vi "Executor_v2.vi"() -> ()   [LabVIEW 2018]
uses:
  QBuilder Files/Actions_arr.ctl
  QBuilder Files/Action.ctl
  QBuilder Files/Parameters.ctl
  Executor Files/MacroInfo.ctl
  Executor Files/Calibrations.ctl
  Executor Files/VariableScan_Cluster.ctl
  Executor Files/RT Actions.ctl
  Executor Files/RT/ActionCluster.ctl
  Executor Files/RT/Instructions_RT.ctl
  Executor Files/RT/ParameterSubCluster.ctl
  Executor Files/State.ctl
  <vilib>/NI/AMC/Message Queue.ctl
  <vilib>/NI/AMC/Message.ctl
  <vilib>/NI/Tools/Keyed Array/KeyedArray.ctl
  Executor Files/RT/Target/Request.ctl
  <vilib>/NI/AMC/Create Single Message.vi
  <vilib>/NI/AMC/Update Message Routing Info.vi
  <vilib>/NI/AMC/Read Termination Message.vi
  <vilib>/NI/AMC/Send Message.vi
  <vilib>/NI/AMC/Globals.vi
  <vilib>/NI/AMC/AMC.lvlib
  <vilib>/NI/Tools/Keyed Array/Tools_KeyedArray.lvlib
panel:
  out "State":T1=enum."idle"
  out "Times (ms)":i64[](array[numeric])
  in  "System":u16(ring)=1 items=["Cusp", "Positron", "Musashi"]
  out "# always zero":i32
  out "error out":errorcluster
  in  "Macro Info 2D":T2(array[cluster])=[[{"Duration (s)"=0.1, "Instruction Description"="", "Input Bits"=[], "Output Bits"=[FALSE, FALSE, FALSE, FALSE, FALSE, FALSE, FALSE, FALSE, FALSE, FALSE, FALSE, FALSE, FALSE, FALSE, FALSE, FALSE, FALSE, FALSE, FALSE, FALSE, FALSE, FALSE, FALSE, FALSE, FALSE, FALSE, FALSE, FALSE, FALSE, FALSE, FALSE, FALSE, FALSE, FALSE, FALSE, FALSE, FALSE, FALSE], "Excitations"=[0.0, 0.0, 0.0, 0.0, 0.0, 0.0, 0.0, 0.0, 0.0, 0.0, 0.0, 0.0, 0.0, 0.0, 0.0, 0.0, 0.0, 0.0, 0.0, 0.0, 0.0, 0.0, 0.0, 0.0], "Steps"=1, "Changes"=[TRUE, TRUE]}, {"Duration (s)"=0.0, "Instruction Description"="", "Input Bits"=[], "Output Bits"=[], "Excitations"=[], "Steps"=0, "Changes"=[]}, {"Duration (s)"=0.0, "Instruction Description"="", "Input Bits"=[], "Output Bits"=[], "Excitations"=[], "Steps"=0, "Changes"=[]}, {"Duration (s)"=0.0, "Instruction Description"="", "Input Bits"=[], "Output Bits"=[], "Excitations"=[], "Steps"=0, "Changes"=[]}], [{"Duration (s)"=0.2, "Instruction Description"="", "Input Bits"=[], "Output Bits"=[FALSE, FALSE, FALSE, FALSE, FALSE, FALSE, FALSE, FALSE, FALSE, FALSE, FALSE, FALSE, FALSE, FALSE, FALSE, FALSE, FALSE, FALSE, FALSE, FALSE, FALSE, FALSE, FALSE, FALSE, FALSE, FALSE, FALSE, FALSE, FALSE, FALSE, FALSE, FALSE, FALSE, FALSE, FALSE, FALSE, FALSE, FALSE], "Excitations"=[0.0, 0.0, 0.0, 0.0, 0.0, 0.0, 0.0, 0.0, 0.0, 0.0, 0.0, 0.0, 0.0, 0.0, 0.0, 0.0, 0.0, 0.0, 0.0, 0.0, 0.0, 0.0, 0.0, 0.0], "Steps"=1, "Changes"=[TRUE, TRUE]}, {"Duration (s)"=0.0, "Instruction Description"="", "Input Bits"=[], "Output Bits"=[], "Excitations"=[], "Steps"=0, "Changes"=[]}, {"Duration (s)"=0.0, "Instruction Description"="", "Input Bits"=[], "Output Bits"=[], "Excitations"=[], "Steps"=0, "Changes"=[]}, {"Duration (s)"=0.0, "Instruction Description"="", "Input Bits"=[], "Output Bits"=[], "Excitations"=[], "Steps"=0, "Changes"=[]}], [{"Duration (s)"=0.3, "Instruction Description"="", "Input Bits"=[], "Output Bits"=[FALSE, FALSE, FALSE, FALSE, FALSE, FALSE, FALSE, FALSE, FALSE, FALSE, FALSE, FALSE, FALSE, FALSE, FALSE, FALSE, FALSE, FALSE, FALSE, FALSE, FALSE, FALSE, FALSE, FALSE, FALSE, FALSE, FALSE, FALSE, FALSE, FALSE, FALSE, FALSE, FALSE, FALSE, FALSE, FALSE, FALSE, FALSE], "Excitations"=[0.0, 0.0, 0.0, 0.0, 0.0, 0.0, 0.0, 0.0, 0.0, 0.0, 0.0, 0.0, 0.0, 0.0, 0.0, 0.0, 0.0, 0.0, 0.0, 0.0, 0.0, 0.0, 0.0, 0.0], "Steps"=1, "Changes"=[TRUE, TRUE]}, {"Duration (s)"=0.0, "Instruction Description"="", "Input Bits"=[], "Output Bits"=[], "Excitations"=[], "Steps"=0, "Changes"=[]}, {"Duration (s)"=0.0, "Instruction Description"="", "Input Bits"=[], "Output Bits"=[], "Excitations"=[], "Steps"=0, "Changes"=[]}, {"Duration (s)"=0.0, "Instruction Description"="", "Input Bits"=[], "Output Bits"=[], "Excitations"=[], "Steps"=0, "Changes"=[]}], [{"Duration (s)"=0.01, "Instruction Description"="", "Input Bits"=[], "Output Bits"=[FALSE, FALSE, FALSE, FALSE, FALSE, FALSE, FALSE, FALSE, FALSE, FALSE, FALSE, FALSE, FALSE, FALSE, FALSE, FALSE, FALSE, FALSE, FALSE, FALSE, FALSE, FALSE, FALSE, FALSE, FALSE, FALSE, FALSE, FALSE, FALSE, FALSE, FALSE, FALSE, FALSE, FALSE, FALSE, FALSE, FALSE, FALSE], "Excitations"=[-0.00023318098842089834, -0.00044019955713256676, -0.0004811194044810927, -0.0003270089360197006, -0.00037474988790963174, -0.00027444024231065297, 0.6717526466140145, -0.0003012834675718561, -0.0003574123346967952, -0.0002612820237967628, -0.00044389144836399103, -0.0003012330472735062, -0.00021413562815348174, -0.000348292029470864, -0.0006236629805725628, -0.0003687933751299158, -0.0009869232667160128, -0.00016073401868532967, -0.000402023518375825, -0.0002482954850485854, -0.0003689863609223317, -0.00026807315716459023, -8.725125004194771e-05, -0.00026778601219765283], "Steps"=1, "Changes"=[TRUE, FALSE]}, {"Duration (s)"=0.02, "Instruction Description"="", "Input Bits"=[], "Output Bits"=[FALSE, FALSE, FALSE, FALSE, FALSE, FALSE, FALSE, FALSE, FALSE, FALSE, FALSE, FALSE, FALSE, FALSE, FALSE, FALSE, FALSE, FALSE, FALSE, FALSE, FALSE, FALSE, FALSE, FALSE, FALSE, FALSE, FALSE, FALSE, FALSE, FALSE, FALSE, FALSE, FALSE, FALSE, FALSE, FALSE, FALSE, FALSE], "Excitations"=[-0.00023318098842089834, -0.00044019955713256676, -0.0004811194044810927, -0.0003270089360197006, -0.00037474988790963174, -0.00027444024231065297, 0.6717526466140145, -0.0003012834675718561, -0.0003574123346967952, -0.0002612820237967628, -0.00044389144836399103, -0.0003012330472735062, -0.00021413562815348174, -0.000348292029470864, -0.0006236629805725628, -0.0003687933751299158, -0.0009869232667160128, -0.00016073401868532967, -0.000402023518375825, -0.0002482954850485854, -0.0003689863609223317, -0.00026807315716459023, -8.725125004194771e-05, -0.00026778601219765283], "Steps"=100, "Changes"=[FALSE, TRUE]}, {"Duration (s)"=0.1, "Instruction Description"="wait", "Input Bits"=[], "Output Bits"=[FALSE, FALSE, FALSE, FALSE, FALSE, FALSE, FALSE, FALSE, FALSE, FALSE, FALSE, FALSE, FALSE, FALSE, FALSE, FALSE, FALSE, FALSE, FALSE, FALSE, FALSE, FALSE, FALSE, FALSE, FALSE, FALSE, FALSE, FALSE, FALSE, FALSE, FALSE, FALSE, FALSE, FALSE, FALSE, FALSE, FALSE, FALSE], "Excitations"=[-0.00023318098842089834, -0.00044019955713256676, -0.0004811194044810927, -0.0003270089360197006, -0.00037474988790963174, -0.00027444024231065297, 0.6717526466140145, -0.0003012834675718561, -0.0003574123346967952, -0.0002612820237967628, -0.00044389144836399103, -0.0003012330472735062, -0.00021413562815348174, -0.000348292029470864, -0.0006236629805725628, -0.0003687933751299158, -0.0009869232667160128, -0.00016073401868532967, -0.000402023518375825, -0.0002482954850485854, -0.0003689863609223317, -0.00026807315716459023, -8.725125004194771e-05, -0.00026778601219765283], "Steps"=1, "Changes"=[FALSE, FALSE]}, {"Duration (s)"=0.01, "Instruction Description"="wait", "Input Bits"=[], "Output Bits"=[FALSE, FALSE, FALSE, FALSE, FALSE, FALSE, FALSE, FALSE, FALSE, FALSE, FALSE, FALSE, FALSE, FALSE, FALSE, FALSE, FALSE, FALSE, FALSE, FALSE, FALSE, FALSE, FALSE, FALSE, FALSE, FALSE, FALSE, FALSE, FALSE, FALSE, FALSE, FALSE, FALSE, FALSE, FALSE, FALSE, FALSE, FALSE], "Excitations"=[-0.00023318098842089834, -0.00044019955713256676, -0.0004811194044810927, -0.0003270089360197006, -0.00037474988790963174, -0.00027444024231065297, -0.0004032935641068728, -0.0003012834675718561, -0.0003574123346967952, -0.0002612820237967628, -0.00044389144836399103, -0.0003012330472735062, -0.00021413562815348174, -0.000348292029470864, -0.0006236629805725628, -0.0003687933751299158, -0.0009869232667160128, -0.00016073401868532967, -0.000402023518375825, -0.0002482954850485854, -0.0003689863609223317, -0.00026807315716459023, -8.725125004194771e-05, -0.00026778601219765283], "Steps"=100, "Changes"=[FALSE, TRUE]}], [{"Duration (s)"=0.1, "Instruction Description"="", "Input Bits"=[], "Output Bits"=[FALSE, FALSE, FALSE, FALSE, FALSE, FALSE, FALSE, FALSE, FALSE, FALSE, FALSE, FALSE, FALSE, FALSE, FALSE, FALSE, FALSE, FALSE, FALSE, FALSE, FALSE, FALSE, FALSE, FALSE, FALSE, FALSE, FALSE, FALSE, FALSE, FALSE, FALSE, FALSE, FALSE, FALSE, FALSE, FALSE, FALSE, FALSE], "Excitations"=[-0.00023318098842089834, -0.00044019955713256676, -0.0004811194044810927, -0.0003270089360197006, -0.00037474988790963174, -0.00027444024231065297, -0.0004032935641068728, -0.0003012834675718561, -0.0003574123346967952, -0.0002612820237967628, -0.00044389144836399103, -0.0003012330472735062, -0.00021413562815348174, -0.000348292029470864, -0.0006236629805725628, -0.0003687933751299158, -0.0009869232667160128, -0.00016073401868532967, -0.000402023518375825, -0.0002482954850485854, -0.0003689863609223317, -0.00026807315716459023, -8.725125004194771e-05, -0.00026778601219765283], "Steps"=1, "Changes"=[TRUE, TRUE]}, {"Duration (s)"=0.0, "Instruction Description"="", "Input Bits"=[], "Output Bits"=[], "Excitations"=[], "Steps"=0, "Changes"=[]}, {"Duration (s)"=0.0, "Instruction Description"="", "Input Bits"=[], "Output Bits"=[], "Excitations"=[], "Steps"=0, "Changes"=[]}, {"Duration (s)"=0.0, "Instruction Description"="", "Input Bits"=[], "Output Bits"=[], "Excitations"=[], "Steps"=0, "Changes"=[]}]] {"Duration (s)" format="%_6p"; "Excitations" format="%_3f"}
  in  "stop":bool
  in  "Tab Control":T3(tab)
  in  "List Cycles":u32
  in  "Cycles":u32
  out "Ping":bool
  out "Sending":bool
  in  "Target stale":bool
  in  "Slave?":bool
  in  "Variable Scan":bool
  in  "Zero All":bool
  out "Time (s)":dbl=0.866 format="%.3f"
  out "% completed":dbl(slide)=1.0 scale=0.0..1.0
  out "Duration (s)":dbl=0.8660000000000001 format="%.3f"
  in  "Stale":bool
  in  "Run":bool
  out "Cue Description":string="a few lines of nothing"
  in  "Cue Path":path=path "C:/CuspControl/Positron/1_Cues/Test/2026-04-21/simple3.q"
  out "Cue Info":T4(array[cluster])=[{"Duration (s)"=0.1, "Action Description"=""}, {"Duration (s)"=0.2, "Action Description"=""}, {"Duration (s)"=0.3, "Action Description"=""}, {"Duration (s)"=0.144, "Action Description"="10 V, 0 V"}, {"Duration (s)"=0.1, "Action Description"=""}] {"Duration (s)" format="%_6p"}
  out "Current\nAction":i32
  in  "ABORT":bool
  in  "Favorites":T5(array[cluster])=[{"Cue Path"=path "C:/CuspControl/Positron/1_Cues/RealBaseline/FPS_1s.q", "Slave"=FALSE, "Cycle"=1, "Completed"=0}, {"Cue Path"=path "C:/CuspControl/Positron/1_Cues/RealBaseline/Stack_v23_mcp_1.q", "Slave"=FALSE, "Cycle"=1, "Completed"=0}, {"Cue Path"=path "C:/CuspControl/Positron/1_Cues/Baseline/Stack_v23_s_100.q", "Slave"=FALSE, "Cycle"=1, "Completed"=0}, {"Cue Path"=path "C:/CuspControl/Positron/1_Cues/Util/BiasModerator.q", "Slave"=FALSE, "Cycle"=1, "Completed"=0}]
  out "Timing":i64[](graph)=[104, 204, 304, 150, 104]
  in  "Skip wait":bool
  in  "Params deadtime (s)":dbl=0.004
  in  "Macro deadtime (s)":dbl=0.006
  out "RepAct#list":i32[](array[numeric])=[0, 1, 2, 3, 4]
  in  "# AO cards":u8=3
  out "# trodes\nin calibr":u8=24
  in  "Save Calibration":bool
  in  "Open Calibration":bool
  in  "Calibrations":T6=[{"Gain"=15.0098, "Offset (V)"=0.0035, "Name"="Vm"}, {"Gain"=14.9932, "Offset (V)"=0.0066, "Name"="in"}, {"Gain"=14.9651, "Offset (V)"=0.0072, "Name"="s1"}, {"Gain"=14.9843, "Offset (V)"=0.0049, "Name"="s2"}, {"Gain"=14.9433, "Offset (V)"=0.0056, "Name"="s3r"}, {"Gain"=14.9395, "Offset (V)"=0.0041, "Name"="s3s"}, {"Gain"=14.8775, "Offset (V)"=0.006, "Name"="s4"}, {"Gain"=14.9361, "Offset (V)"=0.0045, "Name"="g8"}, {"Gain"=15.1086, "Offset (V)"=0.0054, "Name"="e1"}, {"Gain"=14.9264, "Offset (V)"=0.0039, "Name"="c1"}, {"Gain"=14.8685, "Offset (V)"=0.0066, "Name"="c2"}, {"Gain"=14.9386, "Offset (V)"=0.0045, "Name"="c3"}, {"Gain"=14.9438, "Offset (V)"=0.0032, "Name"="c4"}, {"Gain"=14.93, "Offset (V)"=0.0052, "Name"="c5"}, {"Gain"=14.9119, "Offset (V)"=0.0093, "Name"="c6"}, {"Gain"=14.9135, "Offset (V)"=0.0055, "Name"="c7"}, {"Gain"=14.9961, "Offset (V)"=0.0148, "Name"="c8"}, {"Gain"=14.9315, "Offset (V)"=0.0024, "Name"="c9"}, {"Gain"=14.9245, "Offset (V)"=0.006, "Name"="e2"}, {"Gain"=14.9016, "Offset (V)"=0.0037, "Name"="--"}, {"Gain"=14.9057, "Offset (V)"=0.0055, "Name"="--"}, {"Gain"=14.9213, "Offset (V)"=0.004, "Name"="--"}, {"Gain"=14.8995, "Offset (V)"=0.0013, "Name"="--"}, {"Gain"=14.9373, "Offset (V)"=0.004, "Name"="--"}] {"Offset (V)" format="%_6p"; "Gain" format="%_6p"}
  in  "Calibration path":path=path "C:/CuspControl/Positron/Configuration/Calibration/Zz_Gal_to_Area.cal"
  out "# electrodes error":bool=TRUE
  in  "outbits (38)":i32=38
  in  "iswap1_1":i32
  in  "iswap1_2":i32
  in  "iswap2_1":i32
  in  "iswap2_2":i32
  in  "Tab Control 2":T7(tab)=enum."VI Server"
  out "Actions":T8=[{"Toggle"=TRUE, "Open parameter editor"=FALSE, "Open MacroEditor"=FALSE, "Macro path"=path "", "Duration (s)"=0.1, "Parameters"=[{"Status"="Camera", "Name"="state (0,1)", "Value"=0.0, "Changed"=FALSE}, {"Status"="Slave", "Name"="state (0,1)", "Value"=0.0, "Changed"=FALSE}, {"Status"="Wait", "Name"="inbit (0...7)", "Value"=0.0, "Changed"=FALSE}, {"Status"="Coils", "Name"="buncher (A)", "Value"=0.0, "Changed"=FALSE}, {"Status"="Coils", "Name"="michishio (A)", "Value"=0.0, "Changed"=FALSE}, {"Status"="Coils", "Name"="acorn (A)", "Value"=0.0, "Changed"=FALSE}, {"Status"="Coils", "Name"="stacker (A)", "Value"=0.0, "Changed"=FALSE}, {"Status"="Coils", "Name"="T2 + T3 (A)", "Value"=0.0, "Changed"=FALSE}, {"Status"="Coils", "Name"="T4 (A)  ", "Value"=0.0, "Changed"=FALSE}, {"Status"="Coils", "Name"="-------- (A)", "Value"=0.0, "Changed"=FALSE}, {"Status"="RW", "Name"="mode (0-9)", "Value"=0.0, "Changed"=FALSE}, {"Status"="RW", "Name"="f_start (Hz)", "Value"=0.0, "Changed"=FALSE}, {"Status"="RW", "Name"="f_stop (Hz)", "Value"=0.0, "Changed"=FALSE}, {"Status"="RW", "Name"="amplitude (V)", "Value"=0.0, "Changed"=FALSE}, {"Status"="RW", "Name"="phase dif (deg)", "Value"=0.0, "Changed"=FALSE}, {"Status"="RW", "Name"="sweep time (s)", "Value"=0.0, "Changed"=FALSE}, {"Status"="HVpuls1", "Name"="enable (0,1)", "Value"=0.0, "Changed"=FALSE}, {"Status"="HVpuls1", "Name"="amplitude (V)", "Value"=0.0, "Changed"=FALSE}, {"Status"="HVpuls2", "Name"="enable (0,1)", "Value"=0.0, "Changed"=FALSE}, {"Status"="HVpuls2", "Name"="amplitude (V)", "Value"=0.0, "Changed"=FALSE}, {"Status"="HVpuls3", "Name"="enable (0,1)", "Value"=0.0, "Changed"=FALSE}, {"Status"="HVpuls3", "Name"="amplitude (V)", "Value"=0.0, "Changed"=FALSE}, {"Status"="MCP", "Name"="front bias (V)", "Value"=0.0, "Changed"=FALSE}, {"Status"="MCP", "Name"="back bias (V)", "Value"=0.0, "Changed"=FALSE}, {"Status"="MCP", "Name"="phos bias (V)", "Value"=0.0, "Changed"=FALSE}, {"Status"="posdaq", "Name"="mode (1 or 0)", "Value"=0.0, "Changed"=FALSE}], "Comment"="", "Reps"=1}, {"Toggle"=TRUE, "Open parameter editor"=FALSE, "Open MacroEditor"=FALSE, "Macro path"=path "", "Duration (s)"=0.2, "Parameters"=[{"Status"="Camera", "Name"="state (0,1)", "Value"=0.0, "Changed"=FALSE}, {"Status"="Slave", "Name"="state (0,1)", "Value"=0.0, "Changed"=FALSE}, {"Status"="Wait", "Name"="inbit (0...7)", "Value"=0.0, "Changed"=FALSE}, {"Status"="Coils", "Name"="buncher (A)", "Value"=0.0, "Changed"=FALSE}, {"Status"="Coils", "Name"="michishio (A)", "Value"=0.0, "Changed"=FALSE}, {"Status"="Coils", "Name"="acorn (A)", "Value"=0.0, "Changed"=FALSE}, {"Status"="Coils", "Name"="stacker (A)", "Value"=0.0, "Changed"=FALSE}, {"Status"="Coils", "Name"="T2 + T3 (A)", "Value"=0.0, "Changed"=FALSE}, {"Status"="Coils", "Name"="T4 (A)  ", "Value"=0.0, "Changed"=FALSE}, {"Status"="Coils", "Name"="-------- (A)", "Value"=0.0, "Changed"=FALSE}, {"Status"="RW", "Name"="mode (0-9)", "Value"=0.0, "Changed"=FALSE}, {"Status"="RW", "Name"="f_start (Hz)", "Value"=0.0, "Changed"=FALSE}, {"Status"="RW", "Name"="f_stop (Hz)", "Value"=0.0, "Changed"=FALSE}, {"Status"="RW", "Name"="amplitude (V)", "Value"=0.0, "Changed"=FALSE}, {"Status"="RW", "Name"="phase dif (deg)", "Value"=0.0, "Changed"=FALSE}, {"Status"="RW", "Name"="sweep time (s)", "Value"=0.0, "Changed"=FALSE}, {"Status"="HVpuls1", "Name"="enable (0,1)", "Value"=0.0, "Changed"=FALSE}, {"Status"="HVpuls1", "Name"="amplitude (V)", "Value"=0.0, "Changed"=FALSE}, {"Status"="HVpuls2", "Name"="enable (0,1)", "Value"=0.0, "Changed"=FALSE}, {"Status"="HVpuls2", "Name"="amplitude (V)", "Value"=0.0, "Changed"=FALSE}, {"Status"="HVpuls3", "Name"="enable (0,1)", "Value"=0.0, "Changed"=FALSE}, {"Status"="HVpuls3", "Name"="amplitude (V)", "Value"=0.0, "Changed"=FALSE}, {"Status"="MCP", "Name"="front bias (V)", "Value"=0.0, "Changed"=FALSE}, {"Status"="MCP", "Name"="back bias (V)", "Value"=0.0, "Changed"=FALSE}, {"Status"="MCP", "Name"="phos bias (V)", "Value"=0.0, "Changed"=FALSE}, {"Status"="posdaq", "Name"="mode (1 or 0)", "Value"=0.0, "Changed"=FALSE}], "Comment"="", "Reps"=1}, {"Toggle"=TRUE, "Open parameter editor"=FALSE, "Open MacroEditor"=FALSE, "Macro path"=path "", "Duration (s)"=0.3, "Parameters"=[{"Status"="Camera", "Name"="state (0,1)", "Value"=0.0, "Changed"=FALSE}, {"Status"="Slave", "Name"="state (0,1)", "Value"=0.0, "Changed"=FALSE}, {"Status"="Wait", "Name"="inbit (0...7)", "Value"=0.0, "Changed"=FALSE}, {"Status"="Coils", "Name"="buncher (A)", "Value"=0.0, "Changed"=FALSE}, {"Status"="Coils", "Name"="michishio (A)", "Value"=0.0, "Changed"=FALSE}, {"Status"="Coils", "Name"="acorn (A)", "Value"=0.0, "Changed"=FALSE}, {"Status"="Coils", "Name"="stacker (A)", "Value"=0.0, "Changed"=FALSE}, {"Status"="Coils", "Name"="T2 + T3 (A)", "Value"=0.0, "Changed"=FALSE}, {"Status"="Coils", "Name"="T4 (A)  ", "Value"=0.0, "Changed"=FALSE}, {"Status"="Coils", "Name"="-------- (A)", "Value"=0.0, "Changed"=FALSE}, {"Status"="RW", "Name"="mode (0-9)", "Value"=0.0, "Changed"=FALSE}, {"Status"="RW", "Name"="f_start (Hz)", "Value"=0.0, "Changed"=FALSE}, {"Status"="RW", "Name"="f_stop (Hz)", "Value"=0.0, "Changed"=FALSE}, {"Status"="RW", "Name"="amplitude (V)", "Value"=0.0, "Changed"=FALSE}, {"Status"="RW", "Name"="phase dif (deg)", "Value"=0.0, "Changed"=FALSE}, {"Status"="RW", "Name"="sweep time (s)", "Value"=0.0, "Changed"=FALSE}, {"Status"="HVpuls1", "Name"="enable (0,1)", "Value"=0.0, "Changed"=FALSE}, {"Status"="HVpuls1", "Name"="amplitude (V)", "Value"=0.0, "Changed"=FALSE}, {"Status"="HVpuls2", "Name"="enable (0,1)", "Value"=0.0, "Changed"=FALSE}, {"Status"="HVpuls2", "Name"="amplitude (V)", "Value"=0.0, "Changed"=FALSE}, {"Status"="HVpuls3", "Name"="enable (0,1)", "Value"=0.0, "Changed"=FALSE}, {"Status"="HVpuls3", "Name"="amplitude (V)", "Value"=0.0, "Changed"=FALSE}, {"Status"="MCP", "Name"="front bias (V)", "Value"=0.0, "Changed"=FALSE}, {"Status"="MCP", "Name"="back bias (V)", "Value"=0.0, "Changed"=FALSE}, {"Status"="MCP", "Name"="phos bias (V)", "Value"=0.0, "Changed"=FALSE}, {"Status"="posdaq", "Name"="mode (1 or 0)", "Value"=0.0, "Changed"=FALSE}], "Comment"="", "Reps"=1}, {"Toggle"=FALSE, "Open parameter editor"=FALSE, "Open MacroEditor"=FALSE, "Macro path"=path "C:/CuspControl/Positron/1_Macros/Test/2026-04-21/s4.mac", "Duration (s)"=0.144, "Parameters"=[{"Status"="Camera", "Name"="state (0,1)", "Value"=0.0, "Changed"=FALSE}, {"Status"="Slave", "Name"="state (0,1)", "Value"=0.0, "Changed"=FALSE}, {"Status"="Wait", "Name"="inbit (0...7)", "Value"=0.0, "Changed"=FALSE}, {"Status"="Coils", "Name"="buncher (A)", "Value"=0.0, "Changed"=FALSE}, {"Status"="Coils", "Name"="michishio (A)", "Value"=0.0, "Changed"=FALSE}, {"Status"="Coils", "Name"="acorn (A)", "Value"=0.0, "Changed"=FALSE}, {"Status"="Coils", "Name"="stacker (A)", "Value"=0.0, "Changed"=FALSE}, {"Status"="Coils", "Name"="T2 + T3 (A)", "Value"=0.0, "Changed"=FALSE}, {"Status"="Coils", "Name"="T4 (A)  ", "Value"=0.0, "Changed"=FALSE}, {"Status"="Coils", "Name"="-------- (A)", "Value"=0.0, "Changed"=FALSE}, {"Status"="RW", "Name"="mode (0-9)", "Value"=0.0, "Changed"=FALSE}, {"Status"="RW", "Name"="f_start (Hz)", "Value"=0.0, "Changed"=FALSE}, {"Status"="RW", "Name"="f_stop (Hz)", "Value"=0.0, "Changed"=FALSE}, {"Status"="RW", "Name"="amplitude (V)", "Value"=0.0, "Changed"=FALSE}, {"Status"="RW", "Name"="phase dif (deg)", "Value"=0.0, "Changed"=FALSE}, {"Status"="RW", "Name"="sweep time (s)", "Value"=0.0, "Changed"=FALSE}, {"Status"="HVpuls1", "Name"="enable (0,1)", "Value"=0.0, "Changed"=FALSE}, {"Status"="HVpuls1", "Name"="amplitude (V)", "Value"=0.0, "Changed"=FALSE}, {"Status"="HVpuls2", "Name"="enable (0,1)", "Value"=0.0, "Changed"=FALSE}, {"Status"="HVpuls2", "Name"="amplitude (V)", "Value"=0.0, "Changed"=FALSE}, {"Status"="HVpuls3", "Name"="enable (0,1)", "Value"=0.0, "Changed"=FALSE}, {"Status"="HVpuls3", "Name"="amplitude (V)", "Value"=0.0, "Changed"=FALSE}, {"Status"="MCP", "Name"="front bias (V)", "Value"=0.0, "Changed"=FALSE}, {"Status"="MCP", "Name"="back bias (V)", "Value"=0.0, "Changed"=FALSE}, {"Status"="MCP", "Name"="phos bias (V)", "Value"=0.0, "Changed"=FALSE}, {"Status"="posdaq", "Name"="mode (1 or 0)", "Value"=0.0, "Changed"=FALSE}], "Comment"="10 V, 0 V", "Reps"=1}, {"Toggle"=TRUE, "Open parameter editor"=FALSE, "Open MacroEditor"=FALSE, "Macro path"=path "", "Duration (s)"=0.1, "Parameters"=[{"Status"="Camera", "Name"="state (0,1)", "Value"=0.0, "Changed"=FALSE}, {"Status"="Slave", "Name"="state (0,1)", "Value"=0.0, "Changed"=FALSE}, {"Status"="Wait", "Name"="inbit (0...7)", "Value"=0.0, "Changed"=FALSE}, {"Status"="Coils", "Name"="buncher (A)", "Value"=0.0, "Changed"=FALSE}, {"Status"="Coils", "Name"="michishio (A)", "Value"=0.0, "Changed"=FALSE}, {"Status"="Coils", "Name"="acorn (A)", "Value"=0.0, "Changed"=FALSE}, {"Status"="Coils", "Name"="stacker (A)", "Value"=0.0, "Changed"=FALSE}, {"Status"="Coils", "Name"="T2 + T3 (A)", "Value"=0.0, "Changed"=FALSE}, {"Status"="Coils", "Name"="T4 (A)  ", "Value"=0.0, "Changed"=FALSE}, {"Status"="Coils", "Name"="-------- (A)", "Value"=0.0, "Changed"=FALSE}, {"Status"="RW", "Name"="mode (0-9)", "Value"=0.0, "Changed"=FALSE}, {"Status"="RW", "Name"="f_start (Hz)", "Value"=0.0, "Changed"=FALSE}, {"Status"="RW", "Name"="f_stop (Hz)", "Value"=0.0, "Changed"=FALSE}, {"Status"="RW", "Name"="amplitude (V)", "Value"=0.0, "Changed"=FALSE}, {"Status"="RW", "Name"="phase dif (deg)", "Value"=0.0, "Changed"=FALSE}, {"Status"="RW", "Name"="sweep time (s)", "Value"=0.0, "Changed"=FALSE}, {"Status"="HVpuls1", "Name"="enable (0,1)", "Value"=0.0, "Changed"=FALSE}, {"Status"="HVpuls1", "Name"="amplitude (V)", "Value"=0.0, "Changed"=FALSE}, {"Status"="HVpuls2", "Name"="enable (0,1)", "Value"=0.0, "Changed"=FALSE}, {"Status"="HVpuls2", "Name"="amplitude (V)", "Value"=0.0, "Changed"=FALSE}, {"Status"="HVpuls3", "Name"="enable (0,1)", "Value"=0.0, "Changed"=FALSE}, {"Status"="HVpuls3", "Name"="amplitude (V)", "Value"=0.0, "Changed"=FALSE}, {"Status"="MCP", "Name"="front bias (V)", "Value"=0.0, "Changed"=FALSE}, {"Status"="MCP", "Name"="back bias (V)", "Value"=0.0, "Changed"=FALSE}, {"Status"="MCP", "Name"="phos bias (V)", "Value"=0.0, "Changed"=FALSE}, {"Status"="posdaq", "Name"="mode (1 or 0)", "Value"=0.0, "Changed"=FALSE}], "Comment"="", "Reps"=1}] {"Reps" min=1 step=1; "Parameters"."Value" format="%_6p"; "Duration (s)" min=0.001 step=0.001 format="%_6p"}
  out "Insts per Act":i32[](array[numeric])=[1, 1, 1, 4, 1]
  out "RT Actions":T11=[{"Macro Instructions"=[{"Duration (s)"=0.1, "Steps"=1, "Changes"=[TRUE, TRUE], "Triggers"=[FALSE, FALSE, FALSE, FALSE, FALSE, FALSE, FALSE, FALSE, FALSE, FALSE, FALSE, FALSE, FALSE, FALSE, FALSE, FALSE, FALSE, FALSE, FALSE, FALSE, FALSE, FALSE, FALSE, FALSE, FALSE, FALSE, FALSE, FALSE, FALSE, FALSE, FALSE, FALSE, FALSE, FALSE, FALSE, FALSE, FALSE, FALSE], "RAW cmds 2D"=[[0, 0, 0, 0, 0, 0, 0, 0], [0, 0, 0, 0, 0, 0, 0, 0], [0, 0, 0, 0, 0, 0, 0, 0]]}], "Slow AO Array"=[], "Duration (s)"=0.1, "Toggle"=TRUE}, {"Macro Instructions"=[{"Duration (s)"=0.2, "Steps"=1, "Changes"=[TRUE, TRUE], "Triggers"=[FALSE, FALSE, FALSE, FALSE, FALSE, FALSE, FALSE, FALSE, FALSE, FALSE, FALSE, FALSE, FALSE, FALSE, FALSE, FALSE, FALSE, FALSE, FALSE, FALSE, FALSE, FALSE, FALSE, FALSE, FALSE, FALSE, FALSE, FALSE, FALSE, FALSE, FALSE, FALSE, FALSE, FALSE, FALSE, FALSE, FALSE, FALSE], "RAW cmds 2D"=[[0, 0, 0, 0, 0, 0, 0, 0], [0, 0, 0, 0, 0, 0, 0, 0], [0, 0, 0, 0, 0, 0, 0, 0]]}], "Slow AO Array"=[], "Duration (s)"=0.2, "Toggle"=TRUE}, {"Macro Instructions"=[{"Duration (s)"=0.3, "Steps"=1, "Changes"=[TRUE, TRUE], "Triggers"=[FALSE, FALSE, FALSE, FALSE, FALSE, FALSE, FALSE, FALSE, FALSE, FALSE, FALSE, FALSE, FALSE, FALSE, FALSE, FALSE, FALSE, FALSE, FALSE, FALSE, FALSE, FALSE, FALSE, FALSE, FALSE, FALSE, FALSE, FALSE, FALSE, FALSE, FALSE, FALSE, FALSE, FALSE, FALSE, FALSE, FALSE, FALSE], "RAW cmds 2D"=[[0, 0, 0, 0, 0, 0, 0, 0], [0, 0, 0, 0, 0, 0, 0, 0], [0, 0, 0, 0, 0, 0, 0, 0]]}], "Slow AO Array"=[], "Duration (s)"=0.3, "Toggle"=TRUE}, {"Macro Instructions"=[{"Duration (s)"=0.01, "Steps"=1, "Changes"=[TRUE, FALSE], "Triggers"=[FALSE, FALSE, FALSE, FALSE, FALSE, FALSE, FALSE, FALSE, FALSE, FALSE, FALSE, FALSE, FALSE, FALSE, FALSE, FALSE, FALSE, FALSE, FALSE, FALSE, FALSE, FALSE, FALSE, FALSE, FALSE, FALSE, FALSE, FALSE, FALSE, FALSE, FALSE, FALSE, FALSE, FALSE, FALSE, FALSE, FALSE, FALSE], "RAW cmds 2D"=[[0, 0, 0, 0, 0, 0, 0, 0], [0, 0, 0, 0, 0, 0, 0, 0], [0, 0, 0, 0, 0, 0, 0, 0]]}, {"Duration (s)"=0.02, "Steps"=100, "Changes"=[FALSE, TRUE], "Triggers"=[FALSE, FALSE, FALSE, FALSE, FALSE, FALSE, FALSE, FALSE, FALSE, FALSE, FALSE, FALSE, FALSE, FALSE, FALSE, FALSE, FALSE, FALSE, FALSE, FALSE, FALSE, FALSE, FALSE, FALSE, FALSE, FALSE, FALSE, FALSE, FALSE, FALSE, FALSE, FALSE, FALSE, FALSE, FALSE, FALSE, FALSE, FALSE], "RAW cmds 2D"=array3x800[2400 elements]}, {"Duration (s)"=0.1, "Steps"=1, "Changes"=[FALSE, FALSE], "Triggers"=[FALSE, FALSE, FALSE, FALSE, FALSE, FALSE, FALSE, FALSE, FALSE, FALSE, FALSE, FALSE, FALSE, FALSE, FALSE, FALSE, FALSE, FALSE, FALSE, FALSE, FALSE, FALSE, FALSE, FALSE, FALSE, FALSE, FALSE, FALSE, FALSE, FALSE, FALSE, FALSE, FALSE, FALSE, FALSE, FALSE, FALSE, FALSE], "RAW cmds 2D"=[[-1, -1, -2, -1, -1, -1, 2201, -1], [-1, -1, -1, -1, -1, -1, -2, -1], [-3, -1, -1, -1, -1, -1, 0, -1]]}, {"Duration (s)"=0.01, "Steps"=100, "Changes"=[FALSE, TRUE], "Triggers"=[FALSE, FALSE, FALSE, FALSE, FALSE, FALSE, FALSE, FALSE, FALSE, FALSE, FALSE, FALSE, FALSE, FALSE, FALSE, FALSE, FALSE, FALSE, FALSE, FALSE, FALSE, FALSE, FALSE, FALSE, FALSE, FALSE, FALSE, FALSE, FALSE, FALSE, FALSE, FALSE, FALSE, FALSE, FALSE, FALSE, FALSE, FALSE], "RAW cmds 2D"=array3x800[2400 elements]}], "Slow AO Array"=[], "Duration (s)"=0.14, "Toggle"=FALSE}, {"Macro Instructions"=[{"Duration (s)"=0.1, "Steps"=1, "Changes"=[TRUE, TRUE], "Triggers"=[FALSE, FALSE, FALSE, FALSE, FALSE, FALSE, FALSE, FALSE, FALSE, FALSE, FALSE, FALSE, FALSE, FALSE, FALSE, FALSE, FALSE, FALSE, FALSE, FALSE, FALSE, FALSE, FALSE, FALSE, FALSE, FALSE, FALSE, FALSE, FALSE, FALSE, FALSE, FALSE, FALSE, FALSE, FALSE, FALSE, FALSE, FALSE], "RAW cmds 2D"=[[-1, -1, -2, -1, -1, -1, -1, -1], [-1, -1, -1, -1, -1, -1, -2, -1], [-3, -1, -1, -1, -1, -1, 0, -1]]}], "Slow AO Array"=[], "Duration (s)"=0.1, "Toggle"=TRUE}] {"Slow AO Array"."Duration, Gain, NewVal" format="%#_3g"}
  in  "Target IP":string="169.254.48.3"
  in  "Target port":u16=6378
  out "AMC error":errorcluster
  in  "Host port":u16=6674
  in  "GUI_AMCname":string="GUI"
  in  "bite size":i32=5000
  in  "milliseconds to wait":u32=2
  out "RT-to-GUI":T15
  out "Scan-to-GUI":T15
  in  "Scan_AMCname":string="SCAN"
  in  "Scan_AMCname":string="LOCAL"
  out "GUI-to-Scan":T15
  out "PXI card names":string[](array[string])=["DIO:", "6509", "Counter:", "6733_1", "Fast AO:", "6733_1", "6733_2", "6733_3", "Slow AO:", "6723"]
  out "DoDogPaths":string[](array[string])=["C:\\CuspControl\\Positron\\DoDogSubVIs\\SourceCoilControl_Wrapper.vi", "C:\\CuspControl\\GPIB and Network\\SourceCoils.txt", "Source Coils enable (1 or 0)", "1", "C:\\CuspControl\\Positron\\DoDogSubVIs\\RGSBias_Wrapper.vi", "C:\\CuspControl\\GPIB and Network\\RGSBias.txt", "Moderator Bias (V)", "1", "C:\\CuspControl\\Positron\\DoDogSubVIs\\HigakiBSetU-I_Wrapper.vi", "C:\\CuspControl\\GPIB and Network\\HigakiB.txt", "Higaki B charge (1 or 0)", "1", "C:\\CuspControl\\Positron\\DoDogSubVIs\\TLSetAllVoltages_Wrapper.vi", "C:\\CuspControl\\GPIB and Network\\TL.txt", "Transfer Line enable (1 or 0)", "1", "C:\\CuspControl\\Positron\\DoDogSubVIs\\TLSetExitCoil_Wrapper.vi", "C:\\CuspControl\\GPIB and Network\\TL.txt", "Only Extr. Coil enable -> on MCP (1 or 0)", "1", "C:\\CuspControl\\Positron\\DoDogSubVIs\\RGSCoilControl_Wrapper.vi", "C:\\CuspControl\\GPIB and Network\\RGSCoils.txt", "RGS Coils enable (1 or 0)", "1", "C:\\CuspControl\\Positron\\DoDogSubVIs\\HVpulser_Wrapper.vi", "C:\\CuspControl\\GPIB and Network\\HVpulser.txt", "Pulser voltage (divided by 160)", "1"]
  in  "Log Files path":path=path "C:/CuspControl/Positron/Log Files"
  in  "Params paths":path[](array[path])=[path "C:/CuspControl/Cusp/Configuration/Parameters.txt", path "C:/CuspControl/Positron/Configuration/Parameters.txt", path "C:/CuspControl/Musashi/Configuration/Parameters.txt"]
  in  "SlaveState Path":path=path "W:/SlaveState.txt"
  out "Active cue path":path=path "C:/CuspControl/Positron/1_Cues/Test/2026-04-21/simple3.q"
  out "Txt cmds":string[](array[string])=["Action 0\n", "Action 1\n", "Action 2\n", "Action 3\n", "Action 4\n"]
  out "Macro Info (display)":T16=[{"Duration (s)"=0.1, "Instruction Description"="", "Input Bits"=[], "Output Bits"=[FALSE, FALSE, FALSE, FALSE, FALSE, FALSE, FALSE, FALSE, FALSE, FALSE, FALSE, FALSE, FALSE, FALSE, FALSE, FALSE, FALSE, FALSE, FALSE, FALSE, FALSE, FALSE, FALSE, FALSE, FALSE, FALSE, FALSE, FALSE, FALSE, FALSE, FALSE, FALSE, FALSE, FALSE, FALSE, FALSE, FALSE, FALSE], "Excitations"=[0.0035, 0.0066, 0.0072, 0.0049, 0.0056, 0.0041, 0.006, 0.0045, 0.0054, 0.0039, 0.0066, 0.0045, 0.0032, 0.0052, 0.0093, 0.0055, 0.0148, 0.0024, 0.006, 0.0037, 0.0055, 0.004, 0.0013, 0.004], "Steps"=1, "Changes"=[TRUE, TRUE]}, {"Duration (s)"=0.0, "Instruction Description"="", "Input Bits"=[], "Output Bits"=[], "Excitations"=[], "Steps"=0, "Changes"=[]}, {"Duration (s)"=0.0, "Instruction Description"="", "Input Bits"=[], "Output Bits"=[], "Excitations"=[], "Steps"=0, "Changes"=[]}, {"Duration (s)"=0.0, "Instruction Description"="", "Input Bits"=[], "Output Bits"=[], "Excitations"=[], "Steps"=0, "Changes"=[]}] {"Duration (s)" format="%_6p"}
  in  "Variable Cluster":T17={"Values"=[0.10000000000000003, 0.20000000000000004, 0.30000000000000004], "Action"=1, "Inst."=0, "# Elements"=3, "Next Element"=2, "First Val"=0.10000000000000003, "Final Val"=0.30000000000000004, "Update Array"=FALSE, "Description"="", "Variable Type"=0, "Scan Now"=TRUE, "# Act/Inst."=2, "Electrodes_range"=[], "Parameter Name"="RW&f_start (Hz)", "# Passes"=1} {"Variable Type" items=["Duration (s)", "Voltage (V)", "Parameter"]; "Final Val" format="%_6p"; "First Val" format="%_6p"; "Values" format="%_6p"}
  out "Last Modified (when loaded)":timestamp=timestamp(3859615508 s since 1904-01-01)
  # "u13            u12            u11             u10            u9             u8              u7             u6              u5             u4              u3"
  # "swap electrode lines"
  # "swap electrode lines"
  # "0        2       4       6        8      10     12     14"
  # "0        2       4       6        8      10     12     14     16     18      20    22     24     26     28     30     32     34     36"
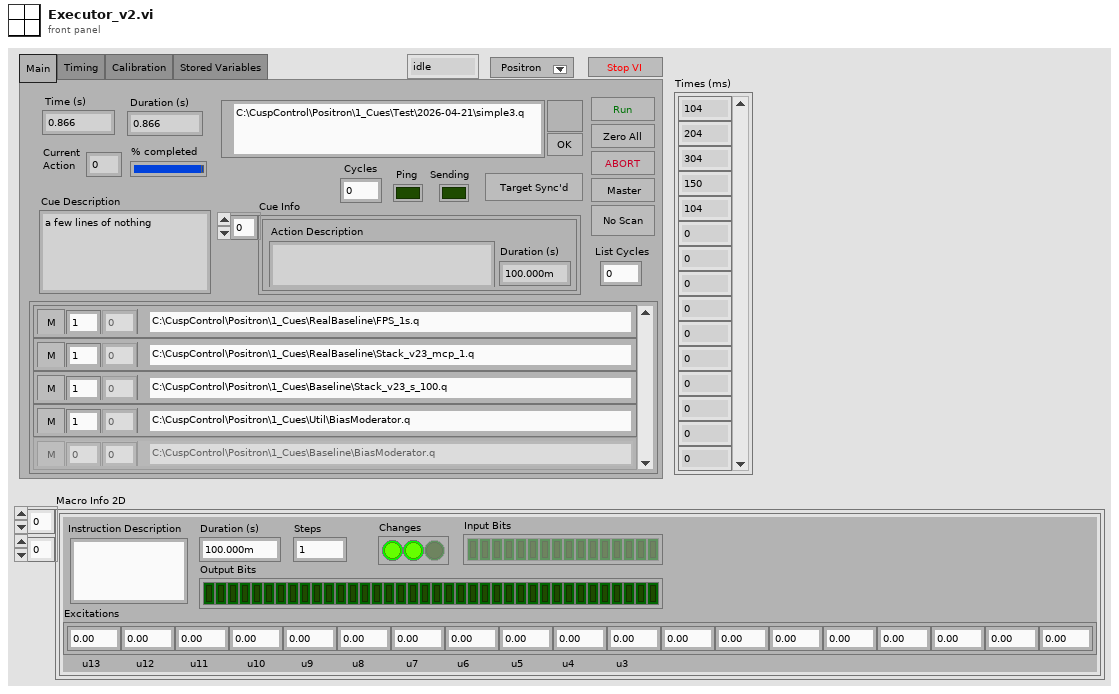
[diagram p1: front panel]
types:
  T1 = typedef "State.ctl" = enum16{"stale", "target stale", "run", "zero all", "open cal", "save cal", "idle"}
  T2 = cluster{"Duration (s)":dbl, "Instruction Description":string, "Input Bits":bool[], "Output Bits":bool[], "Excitations":dbl[], "Steps":i32, "Changes":bool[]}[][]
  T3 = enum32{"Main", "Timing", "Calibration", "Stored Variables"}
  T4 = cluster{"Duration (s)":dbl, "Action Description":string}[]
  T5 = cluster{"Cue Path":path, "Slave":bool, "Cycle":u32, "Completed":u32}[]
  T6 = typedef "Calibrations.ctl" = cluster{"Gain":dbl, "Offset (V)":dbl, "Name":string}[]
  T7 = enum32{"Actions", "RT Actions", "VI Server", "Paths and names", "Text commands", "old display", "variable cluster"}
  T8 = typedef "Actions_arr.ctl" = T9[]
  T9 = typedef "Action.ctl" = cluster{"Toggle":bool, "Open parameter editor":bool, "Open MacroEditor":bool, "Macro path":path, "Duration (s)":dbl, "Parameters":T10, "Comment":string, "Reps":i32}
  T10 = typedef "Parameters.ctl" = cluster{"Status":string, "Name":string, "Value":dbl, "Changed":bool}[]
  T11 = typedef "RT Actions.ctl" = T12[]
  T12 = typedef "ActionCluster.ctl" = cluster{"Macro Instructions":T13, "Slow AO Array":T14, "Duration (s)":dbl, "Toggle":bool}
  T13 = typedef "Instructions_RT.ctl" = cluster{"Duration (s)":dbl, "Steps":i32, "Changes":bool[], "Triggers":bool[], "RAW cmds 2D":i16[][]}[]
  T14 = typedef "ParameterSubCluster.ctl" = cluster{"ao line":string, "Duration, Gain, NewVal":dbl[]}[]
  T15 = typedef "AMC.lvlib/Message Queue.ctl" = refnum<queue>
  T16 = typedef "MacroInfo.ctl" = cluster{"Duration (s)":dbl, "Instruction Description":string, "Input Bits":bool[], "Output Bits":bool[], "Excitations":dbl[], "Steps":i32, "Changes":bool[]}[]
  T17 = typedef "VariableScan_Cluster.ctl" = cluster{"Values":dbl[], "Action":i32, "Inst.":i32, "# Elements":i32, "Next Element":i32, "First Val":dbl, "Final Val":dbl, "Update Array":bool, "Description":string, "Variable Type":u16, "Scan Now":bool, "# Act/Inst.":i32, "Electrodes_range":i32[], "Parameter Name":string, "# Passes":i32}
  T18 = enum32{"Invalid", "Standard", "Closed", "Hidden", "Minimized", "Maximized"}
  T19 = enum8{"Enabled", "Disabled", "Disabled and Grayed Out"}
  T20 = enum16{"open", "replace", "create", "open or create", "replace or create", "replace or create with confirmation"}
  T21 = typedef "Request.ctl" = enum16{"Start", "Run", "Skip Wait", "Pause", "Unpause", "Abort", "Shutdown"}
  T22 = cluster{"Cue Path":path, "Slave":bool, "Cycle":u32, "Completed":u32}
  T23 = cluster{"Total\nTime (s)":dbl, "Cue Description":string}
  T24 = cluster{"Duration (s)":dbl, "Action Description":string}
  T25 = cluster{"Duration (s)":dbl, "Instruction Description":string, "Input Bits":bool[], "Output Bits":bool[], "Excitations":dbl[], "Steps":i32, "Changes":bool[]}
  T26 = typedef "MacroSaveCluster.ctl" = cluster{"Instructions":T27, "Changes":bool[][], "Macro Description":string, "Total Time (s)":dbl, "Samples per sec":dbl}
  T27 = typedef "Instructions.ctl" = T28[]
  T28 = typedef "Instruction.ctl" = cluster{"Duration":dbl, "Comment":string, "Steps":i32, "Edit Potential":bool, "Output Bits":bool[], "Macro Path":path, "Potentials":dbl[], "Inherit?":bool}
  T29 = cluster{"Duration (s)":dbl, "Instruction Description":string, "Input Bits":bool[], "Output Bits":bool[], "Excitations":dbl[], "Steps":i32, "Changes":bool[]}[]
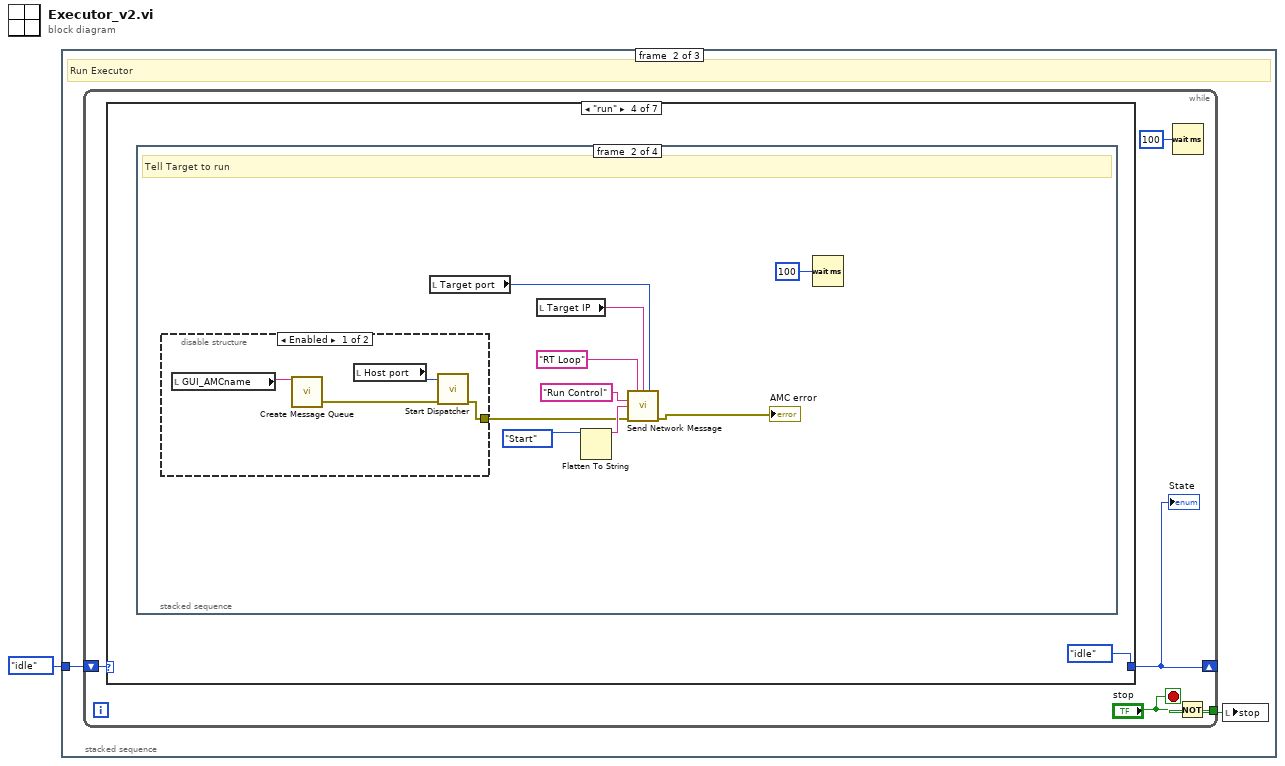
[diagram p0: block diagram]
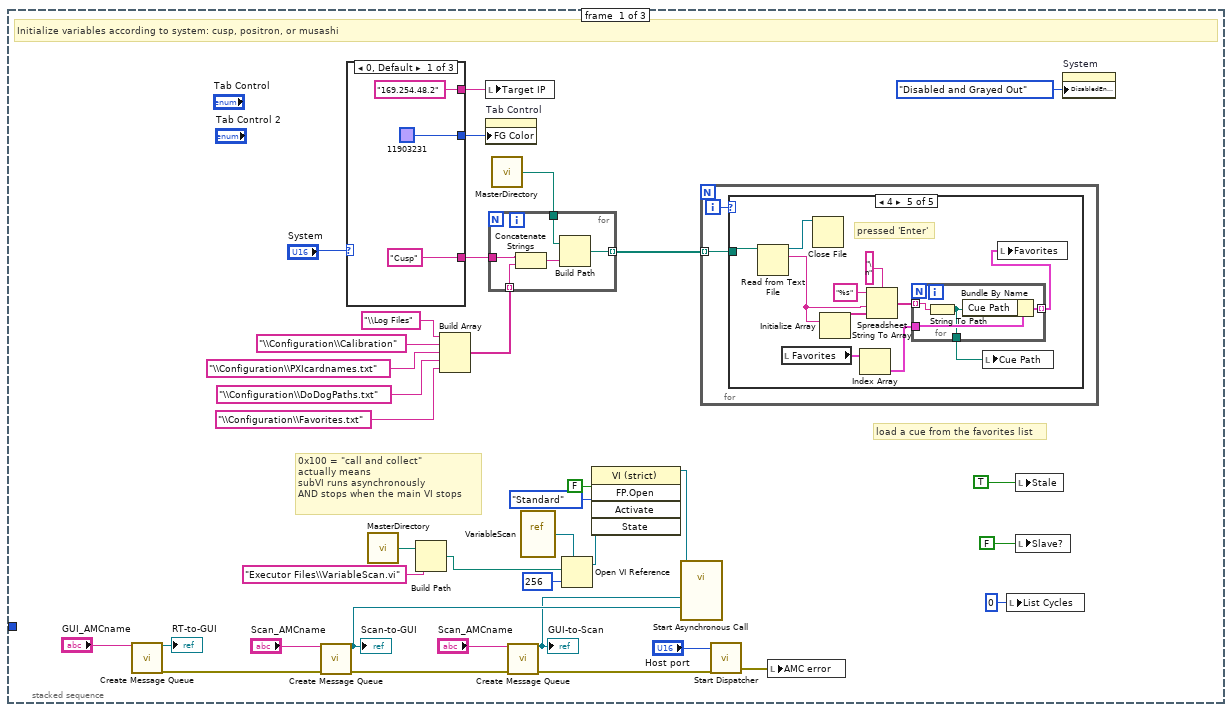
[diagram p2: hidden frame]
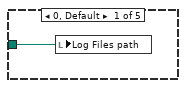
[diagram p3: hidden frame]
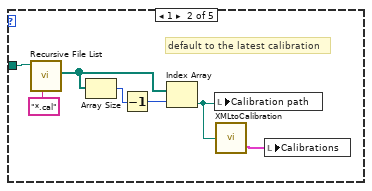
[diagram p4: hidden frame]
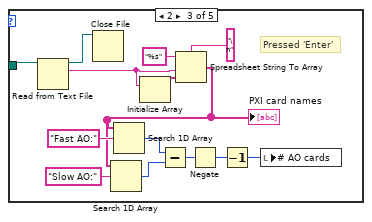
[diagram p5: hidden frame]
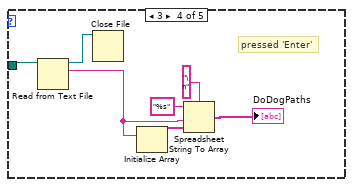
[diagram p6: hidden frame]
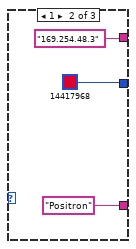
[diagram p7: hidden frame]
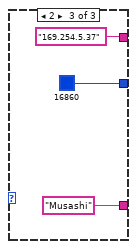
[diagram p8: hidden frame]
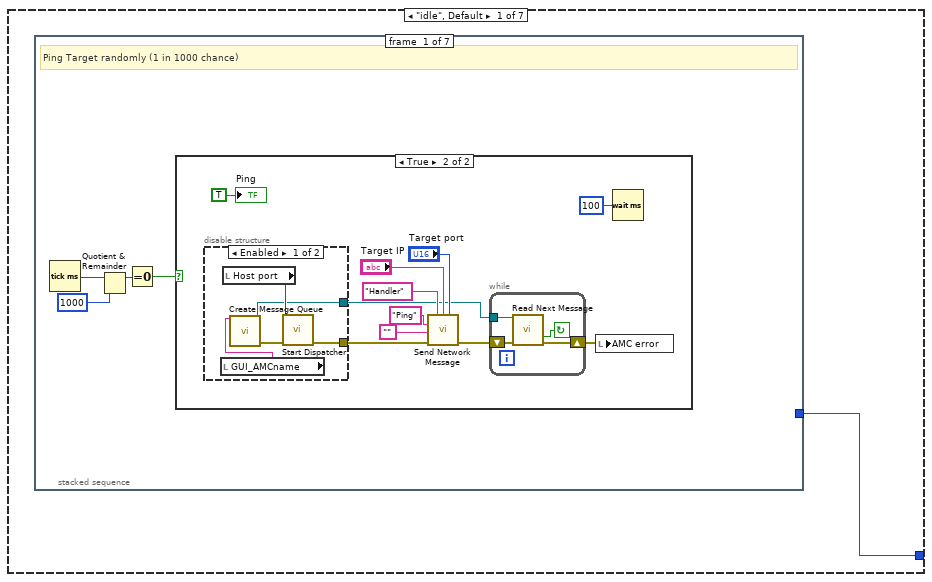
[diagram p9: hidden frame]
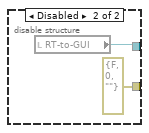
[diagram p11: hidden frame]
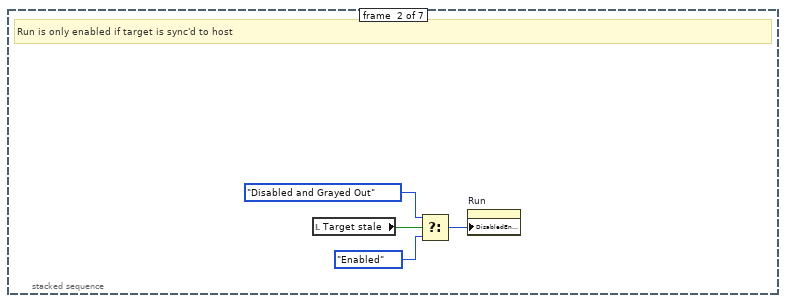
[diagram p12: hidden frame]
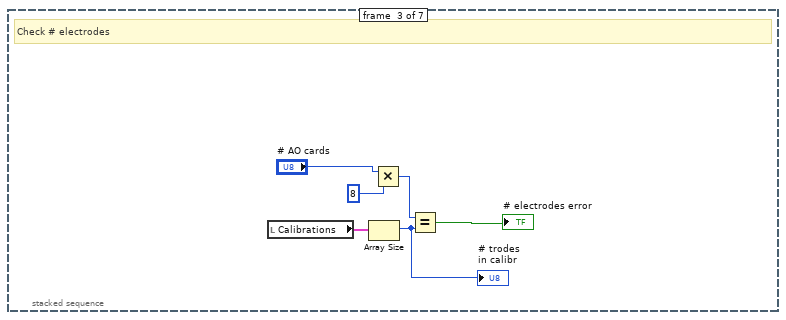
[diagram p13: hidden frame]
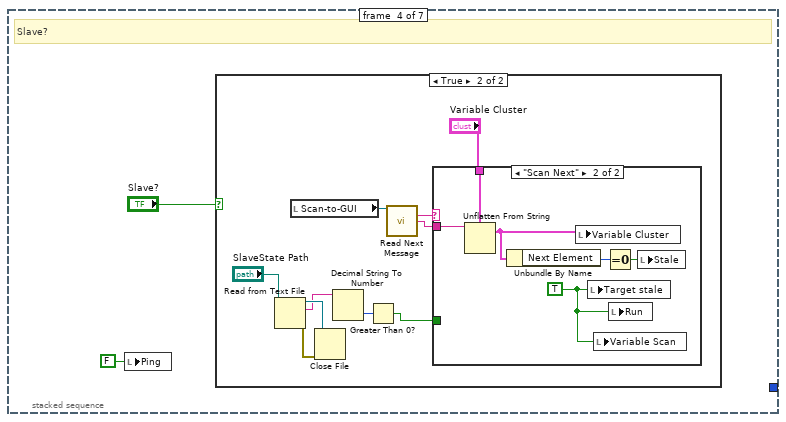
[diagram p14: hidden frame]
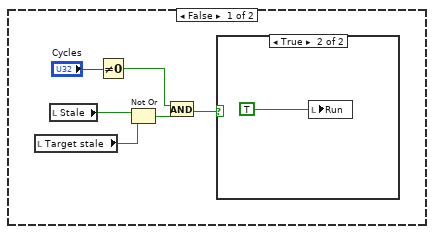
[diagram p15: hidden frame]
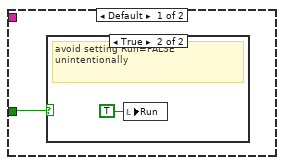
[diagram p17: hidden frame]
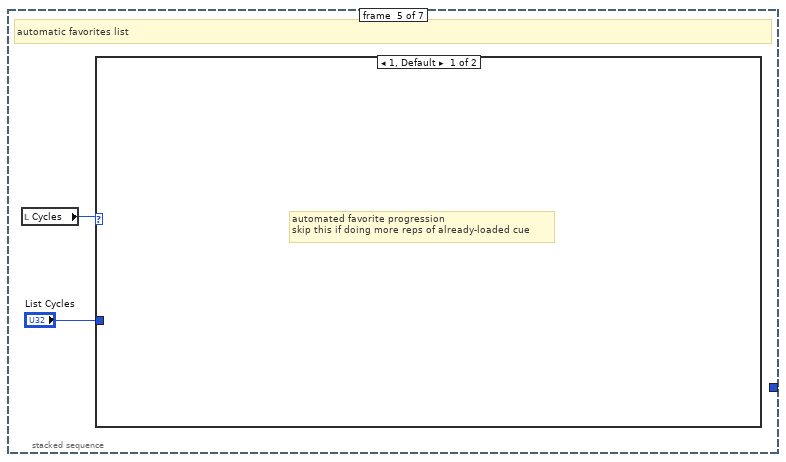
[diagram p19: hidden frame]
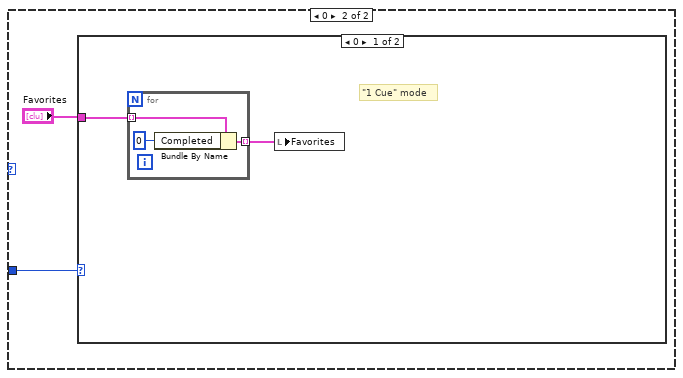
[diagram p20: hidden frame]
diagram:
  n1 = stacked-sequence {
    tunnel: State."idle" ("State") -> [_ w98 _]
    frame #0 {
      # "0x100 = \"call and collect\" \nactually means\nsubVI runs asynchronously\nAND stops when the main VI stops"
      # "load a cue from the favorites list"
      # "Initialize variables according to system: cusp, positron, or musashi"
      n2 = call <vilib>:"Create Message Queue.vi"("message queue name"="GUI_AMCname") -> ("message queue out"=→"RT-to-GUI":T15, "error out"=w17:errorcluster)  [unwired: 13 in]
      n3 = call <vilib>:"Create Message Queue.vi"("message queue name"="Scan_AMCname", "error in"=w17) -> ("message queue out"=w10:T15, "error out"=w13:errorcluster)  [unwired: 12 in]
      "Scan-to-GUI" <- w10
      n4 = case shown="0, Default" "System" {
        tunnel: ["Cusp" ("string") "Positron" ("string") "Musashi" ("string")] -> w33
        tunnel: [u32 11903231 u32 14417968 u32 16860] -> w28
        tunnel: ["169.254.48.2" ("Target IP") "169.254.48.3" ("Target IP") "169.254.5.37" ("Target IP")] -> w27
        frame 0, Default {
        }
        frame 1 {
        }
        frame 2 {
        }
      }
      n5 = call "MasterDirectory.vi"() -> ("Master Directory"=w7:path)
      n6 = Build Path(base path=w7, name or relative path="Executor Files\\VariableScan.vi") -> (appended path=w6:path)
      n7 = Build Array("\\Log Files", "\\Configuration\\Calibration", "\\Configuration\\PXIcardnames.txt", "\\Configuration\\DoDogPaths.txt", "\\Configuration\\Favorites.txt") -> (w32:string[])
      n8 = local write "Target IP"(w27) -> ()
      n9 = property on="Tab Control" class="TabCtl (strict)"("FG Color"=w28) -> ()  [unwired: 2 in, 2 out]
      n10 = call "MasterDirectory.vi"() -> ("Master Directory"=w30:path)
      n11 = for {
        tunnel: w33 -> [w87]
        tunnel: w30 -> [w84]
        tunnel: w32 -> [w86] mode=indexing
        tunnel: [w85] -> w29 mode=indexing
        n12 = Concatenate Strings(w87, w86) -> (w88:string)
        n13 = Build Path(base path=w84, name or relative path=w88) -> (appended path=w85:path)
      }
      n14 = call <vilib>:"Create Message Queue.vi"("message queue name"="Scan_AMCname", "error in"=w13) -> ("message queue out"=w9:T15, "error out"=w16:errorcluster)  [unwired: 12 in]
      "GUI-to-Scan" <- w9
      n15 = vi-ref "VariableScan.vi"() -> (w12:refnum<vi>)
      n16 = Open VI Reference(type specifier VI Refnum (for type only)=w12, vi path=w6, options=256) -> (vi reference=w5:refnum<vi>)  [unwired: 3 in, 1 out]
      n17 = invoke class="VI (strict)" method="FP.Open"(reference=w5, "Activate"=FALSE ("Activate?"), "State"=T18."Standard") -> (reference out=w2:refnum<vi>)  [unwired: 2 in, 4 out]
      n18 = call-by-ref "Start Asynchronous Call"(reference=w2, "Scan-to-GUI"=w10, "GUI-to-Scan"=w9) -> ()  [unwired: 2 in, 2 out]
      n19 = for {
        tunnel: w29 -> [w38] mode=indexing
        i -> [w39]
        n20 = case shown="4" w39 {
          tunnel: w38 -> [w40 w42 w57 w64 w75]
          frame 0, Default {
            n21 = local write "Log Files path"(w40) -> ()
          }
          frame 1 {
            # "default to the latest calibration"
            n22 = call <vilib>:"Recursive File List.vi"("pattern"="*.cal", "Folder Path"=w42) -> ("All Files in Dir"=w41:path[])  [unwired: 5 in, 4 out]
            n23 = Array Size(array=w41) -> (size(s)=w45:i32)
            n24 = Decrement(x=w45) -> (x-1=w44:i32)
            n25 = Index Array(array=w41, index=w44) -> (element=w47:path)
            n26 = local write "Calibration path"(w47) -> ()
            n27 = call "XMLtoCalibration.vi"("XML File Path"=w47) -> ("Calibrations"=w46:T6)  [unwired: 1 in]
            n28 = local write "Calibrations"(w46) -> ()
          }
          frame 2 {
            # "Pressed 'Enter'"
            n29 = Read from Text File(file (use dialog)=w57) -> (refnum out=w61:refnum<file>, text=w59:string)  [unwired: 3 in, 2 out]
            n30 = Close File(refnum=w61) -> ()  [unwired: 1 in, 2 out]
            n31 = Initialize Array(w59) -> (w60:string[])  [unwired: 1 in]
            n32 = Spreadsheet String To Array(delimiter (Tab)="\n", format string="%s", spreadsheet string=w59, array type (2D Dbl)=w60) -> (array=w55:string[])
            "PXI card names" <- w55
            n33 = Search 1D Array(1D array=w55, element="Slow AO:") -> (index of element=w52:i32)  [unwired: 1 in]
            n34 = Search 1D Array(1D array=w55, element="Fast AO:") -> (index of element=w53:i32)  [unwired: 1 in]
            n35 = Subtract(x=w53, y=w52) -> (x-y=w51:i32)
            n36 = Negate(x=w51) -> (-x=w50:i32)
            n37 = Decrement(x=w50) -> (x-1=w49:i32)
            n38 = local write "# AO cards"(w49) -> ()
          }
          frame 3 {
            # "pressed 'Enter'"
            n39 = Read from Text File(file (use dialog)=w64) -> (refnum out=w68:refnum<file>, text=w66:string)  [unwired: 3 in, 2 out]
            n40 = Close File(refnum=w68) -> ()  [unwired: 1 in, 2 out]
            n41 = Initialize Array(w66) -> (w67:string[])  [unwired: 1 in]
            n42 = Spreadsheet String To Array(delimiter (Tab)="\n", format string="%s", spreadsheet string=w66, array type (2D Dbl)=w67) -> (array=→"DoDogPaths":string[])
          }
          frame 4 {
            # "pressed 'Enter'"
            n43 = Read from Text File(file (use dialog)=w75) -> (refnum out=w79:refnum<file>, text=w77:string)  [unwired: 3 in, 2 out]
            n44 = local read "Favorites"() -> (w73:T5)
            n45 = Close File(refnum=w79) -> ()  [unwired: 1 in, 2 out]
            n46 = Initialize Array(w77) -> (w78:string[])  [unwired: 1 in]
            n47 = Index Array(array=w73) -> (element=w72:T22)  [unwired: 1 in]
            n48 = Spreadsheet String To Array(delimiter (Tab)="\n", format string="%s", spreadsheet string=w77, array type (2D Dbl)=w78) -> (array=w71:string[])
            n49 = for {
              tunnel: w72 -> [w83]
              tunnel: w71 -> [w81] mode=indexing
              tunnel: [w82] -> w70 mode=indexing
              tunnel: [w80] -> w69
              n50 = String To Path(string=w81) -> (path=w80:path)
              n51 = Bundle By Name(cluster=w83, "Cue Path"=w80) -> (w82:T22)
            }
            n52 = local write "Cue Path"(w69) -> ()
            n53 = local write "Favorites"(w70) -> ()
          }
        }
      }
      n54 = call <vilib>:"Start Dispatcher.vi"("UDP port (0)"="Host port", "error in"=w16) -> ("error out"=w20:errorcluster)  [unwired: 11 in, 2 out]
      n55 = local write "AMC error"(w20) -> ()
      n56 = local write "List Cycles"(u32 0 ("List Cycles")) -> ()
      n57 = local write "Stale"(TRUE ("Target stale")) -> ()
      n58 = local write "Slave?"(FALSE ("Target stale")) -> ()
      n59 = property on="System" class="Ring (strict)"("DisabledEnum"=T19."Disabled and Grayed Out" ("Disabled")) -> ()  [unwired: 2 in, 2 out]
    }
    frame #1 {
      # "Run Executor"
      n60 = while {
        tunnel: [w104] -> w99
        shift-right: [w101] -> _
        shift-left: w98 -> [w102]
        stop <- "stop" stop-if-true
        n61 = case shown="\"run\"" w102 {
          tunnel: [w105 State."target stale" ("State") w382 State."idle" ("State") State."idle" ("State") State."stale" ("State") State."idle" ("State")] -> w101
          frame "idle", Default {
            n62 = stacked-sequence {
              tunnel: [_ _ _ _ _ _ w229] -> w105
              frame #0 {
                # "Ping Target randomly (1 in 1000 chance)"
                n63 = Tick Count (ms)() -> (millisecond timer value=w109:u32)
                n64 = Quotient & Remainder(x=w109, y=u32 1000) -> (x-y*floor(x/y)=w107:u32)  [unwired: 1 out]
                n65 = Equal To 0?(x=w107) -> (x = 0?=w106:bool)
                n66 = case shown="True" w106 {
                  frame False {
                  }
                  frame True {
                    n67 = disable-structure shown="Enabled" {
                      disable-tunnel: [w123 errorcluster {"status"=FALSE, "code"=0, "source"=""} ("error in")] -> w112
                      disable-tunnel: [w122 w127] -> w110
                      frame Enabled {
                        n68 = local read "GUI_AMCname"() -> (w121:string)
                        n69 = local read "Host port"() -> (w124:u16)
                        n70 = call <vilib>:"Create Message Queue.vi"("message queue name"=w121) -> ("message queue out"=w122:T15, "error out"=w125:errorcluster)  [unwired: 13 in]
                        n71 = call <vilib>:"Start Dispatcher.vi"("UDP port (0)"=w124, "error in"=w125) -> ("error out"=w123:errorcluster)  [unwired: 11 in, 2 out]
                      }
                      frame Disabled {
                        n72 = local read "RT-to-GUI"() -> (w127:T15)
                      }
                    }
                    n73 = call <vilib>:"Send Network Message.vi"("receiver process"="Handler", "receiver host"="Target IP", "receiver port (0)"="Target port", "message name"="Ping" ("String"), "message value"="", "error in"=w112) -> ("error out"=w111:errorcluster)  [unwired: 7 in, 2 out]
                    n74 = while {
                      shift-right: [w130] -> w113
                      shift-left: w111 -> [w131]
                      tunnel: w110 -> [w128]
                      stop <- w129 continue-if-true
                      n75 = call <vilib>:"Read Next Message.vi"("message queue in"=w128, "error in"=w131) -> ("timed out?"=w129:bool, "error out"=w130:errorcluster)  [unwired: 6 in, 6 out]
                    }
                    n76 = local write "AMC error"(w113) -> ()
                    n77 = Wait (ms)(milliseconds to wait=u32 100) -> ()  [unwired: 1 out]
                    "Ping" <- TRUE ("Ping")
                  }
                }
              }
              frame #1 {
                # "Run is only enabled if target is sync'd to host"
                n78 = local read "Target stale"() -> (w132:bool)
                n79 = Select(t=T19."Disabled and Grayed Out" ("Disabled"), s=w132, f=T19."Enabled" ("Disabled")) -> (s? t:f=w135:T19)
                n80 = property on="Run" class="Bool (strict)"("DisabledEnum"=w135) -> ()  [unwired: 2 in, 2 out]
              }
              frame #2 {
                # "Check # electrodes"
                n81 = local read "Calibrations"() -> (w141:T6)
                n82 = Array Size(array=w141) -> (size(s)=w136:i32)
                "# trodes\nin calibr" <- w136
                n83 = Multiply(x="# AO cards", y=u8 8) -> (x*y=w139:u8)
                n84 = Equal?(x=w139, y=w136) -> (x = y?=→"# electrodes error":bool)
              }
              frame #3 {
                # "Slave?"
                n85 = local write "Ping"(FALSE ("Ping")) -> ()
                n86 = case shown="True" "Slave?" {
                  frame False {
                    n87 = local read "Target stale"() -> (w148:bool)
                    n88 = local read "Stale"() -> (w144:bool)
                    n89 = Not Equal To 0?(x="Cycles") -> (x != 0?=w146:bool)
                    n90 = Not Or(1:w148, 2:w144) -> (0:w147:bool)
                    n91 = And(x=w146, y=w147) -> (x .and. y?=w145:bool)
                    n92 = case shown="True" w145 {
                      frame False {
                      }
                      frame True {
                        n93 = local write "Run"(TRUE ("Value (Signaling)")) -> ()
                      }
                    }
                  }
                  frame True {
                    n94 = Read from Text File(file (use dialog)="SlaveState Path") -> (refnum out=w159:refnum<file>, text=w157:string, error out=w158:errorcluster)  [unwired: 3 in, 1 out]
                    n95 = local read "Scan-to-GUI"() -> (w153:T15)
                    n96 = Close File(refnum=w159, error in=w158) -> ()  [unwired: 2 out]
                    n97 = Decimal String To Number(string=w157) -> (number=w156:i32)  [unwired: 2 in, 1 out]
                    n98 = Greater Than 0?(x=w156) -> (x > 0?=w155:bool)
                    n99 = call <vilib>:"Read Next Message.vi"("message queue in"=w153) -> ("message name"=w152:string, "message value"=w151:string)  [unwired: 7 in, 6 out]
                    n100 = case shown="\"Scan Next\"" w152 {
                      tunnel: "Variable Cluster" -> [_ w168]
                      tunnel: w155 -> [w161 _]
                      tunnel: w151 -> [_ w167]
                      frame Default {
                        n101 = case shown="True" w161 {
                          frame False {
                          }
                          frame True {
                            # "avoid setting Run=FALSE \nunintentionally"
                            n102 = local write "Run"(TRUE ("Run")) -> ()
                          }
                        }
                      }
                      frame "Scan Next" {
                        w166 = TRUE ("Value (Signaling)")
                        n103 = Unflatten From String(type=w168, binary string=w167) -> (value=w165:T17)  [unwired: 3 in, 2 out]
                        n104 = Unbundle By Name(w165) -> ("Next Element"=w163:i32)
                        n105 = local write "Variable Cluster"(w165) -> ()
                        n106 = local write "Target stale"(w166) -> ()
                        n107 = local write "Variable Scan"(w166) -> ()
                        n108 = Equal To 0?(x=w163) -> (x = 0?=w164:bool)
                        n109 = local write "Run"(w166) -> ()
                        n110 = local write "Stale"(w164) -> ()
                      }
                    }
                  }
                }
              }
              frame #4 {
                # "automatic favorites list"
                n111 = local read "Cycles"() -> (w170:u32)
                n112 = case shown="1, Default" w170 {
                  tunnel: "List Cycles" -> [_ w172]
                  frame 1, Default {
                    # "automated favorite progression\nskip this if doing more reps of already-loaded cue"
                  }
                  frame 0 {
                    n113 = case shown="0" w172 {
                      selector: w172 -> [_ w178]
                      tunnel: "Favorites" -> [w173 w179]
                      frame 0 {
                        # "\"1 Cue\" mode"
                        n114 = for {
                          tunnel: w173 -> [w176] mode=indexing
                          tunnel: [w175] -> w174 mode=indexing
                          n115 = Bundle By Name(cluster=w176, "Completed"=u32 0) -> (w175:T22)
                        }
                        n116 = local write "Favorites"(w174) -> ()
                      }
                      frame 1, Default {
                        n117 = for {
                          tunnel: w179 -> [w204] mode=indexing
                          tunnel: [w204] -> w182
                          tunnel: [w203] -> w181
                          tunnel: [w200] -> w180
                          i -> [w203]
                          stop <- w200 stop-if-true
                          n118 = Unbundle By Name(w204) -> ("Cycle"=w202:u32, "Completed"=w201:u32)
                          n119 = Greater?(x=w202, y=w201) -> (0:w200:bool)
                        }
                        n120 = case shown="False" w180 {
                          tunnel: w179 -> [w186 w199]
                          tunnel: w182 -> [_ w197]
                          tunnel: w181 -> [_ w198]
                          tunnel: w178 -> [w183 _]
                          frame False {
                            # "if last value is false\nthen all cycles have completed\nso go back to the beginning"
                            n121 = for {
                              tunnel: w186 -> [w188] mode=indexing
                              tunnel: [w187] -> w185 mode=indexing
                              n122 = Bundle By Name(cluster=w188, "Completed"=u32 0) -> (w187:T22)
                            }
                            n123 = Decrement(x=w183) -> (x-1=w184:u32)
                            n124 = local write "List Cycles"(w184) -> ()
                            n125 = local write "Favorites"(w185) -> ()
                          }
                          frame True {
                            n126 = Unbundle By Name(w197) -> ("Cue Path"=w193:path, "Slave"=w192:bool)
                            n127 = Unbundle By Name(w197) -> ("Completed"=w195:u32)
                            n128 = Increment(x=w195) -> (x+1=w194:u32)
                            n129 = local write "Cue Path"(w193) -> ()
                            n130 = local write "Slave?"(w192) -> ()
                            n131 = local write "Cycles"(u32 1 ("Cycles")) -> ()
                            n132 = Bundle By Name(cluster=w197, "Completed"=w194) -> (w196:T22)
                            n133 = Replace Array Subset(array=w199, new element=w196, index=w198) -> (w190:T5)
                            n134 = local write "Favorites"(w190) -> ()
                          }
                        }
                      }
                    }
                  }
                }
              }
              frame #5 {
                # "Check for stale"
                n135 = Empty String/Path?(string/path="Cue Path") -> (empty?=w208:bool)
                n136 = call <vilib>:"Check if File or Folder Exists.vi"("path"="Cue Path") -> ("file or folder exists?"=w206:bool, "dup path"=w210:path)  [unwired: 8 in, 1 out]
                n137 = Not(x=w208) -> (.not. x?=w207:bool)
                n138 = And(x=w206, y=w207) -> (x .and. y?=w205:bool)
                n139 = case shown="True" w205 {
                  tunnel: w210 -> [_ w223]
                  frame False {
                    w211 = u32 0 ("List Cycles")
                    n140 = local read "Favorites"() -> (w216:T5)
                    n141 = Array Size(array=w216) -> (size(s)=w213:i32)
                    n142 = Random Number (0-1)() -> (number: 0 to 1=w215:dbl)
                    n143 = Decrement(x=w213) -> (x-1=w212:i32)
                    n144 = Multiply(x=w212, y=w215) -> (x*y=w218:dbl)
                    n145 = Index Array(array=w216, index=w218) -> (element=w217:T22)
                    n146 = One Button Dialog(message="Invalid path.\nLoading another path from the 'favorites' list") -> ()  [unwired: 1 in, 1 out]
                    n147 = Unbundle By Name(w217) -> ("Cue Path"=w214:path)
                    n148 = local write "List Cycles"(w211) -> ()
                    n149 = local write "Cycles"(w211) -> ()
                    n150 = local write "Cue Path"(w214) -> ()
                  }
                  frame True {
                    n151 = local read "Active cue path"() -> (w224:path)
                    n152 = local read "Last Modified (when loaded)"() -> (w226:timestamp)
                    n153 = File/Directory Info(path=w223) -> (last mod=w225:timestamp, error out=w227:errorcluster)  [unwired: 1 in, 5 out]
                    n154 = Not Equal?(x=w223, y=w224) -> (x != y?=w220:bool)
                    n155 = local write "error out"(w227) -> ()
                    n156 = Not Equal?(x=w226, y=w225) -> (x != y?=w221:bool)
                    n157 = Or(x=w221, y=w220) -> (x .or. y?=w222:bool)
                    n158 = case shown="True" w222 {
                      frame False {
                      }
                      frame True {
                        n159 = local write "Stale"(TRUE ("Stale")) -> ()
                      }
                    }
                  }
                }
              }
              frame #6 {
                # ">> Enum >>"
                # ">> Enum Def >>\n                       V\n                       V"
                # ">> Numeric >>"
                # "update state"
                n160 = Build Array("Stale", "Target stale", "Run", "Zero All", "Open Calibration", "Save Calibration", TRUE ("element")) -> (w236:bool[])
                n161 = for {
                  tunnel: w236 -> [w242] mode=indexing
                  tunnel: [w241] -> w230
                  i -> [w241]
                  stop <- w242 stop-if-true
                }
                n162 = To Variant(anything=w230) -> (Variant=w232:variant)
                n163 = Variant To Data(type=State."stale" ("State"), Variant=w232) -> (data=w229:T1)  [unwired: 1 in, 1 out]
              }
            }
          }
          frame "stale" {
            # "This is the only time that the cue \n(and macros) should be opened from disk"
            n164 = local read "# AO cards"() -> (w250:u8)
            n165 = local write "Stale"(FALSE ("Value (Signaling)")) -> ()
            n166 = Multiply(x=w250, y=u8 8) -> (x*y=w249:u8)
            n167 = Initialize Array(0.0 ("element"), w249) -> (w248:dbl[])
            n168 = Initialize Array(FALSE, "outbits (38)") -> (w251:bool[])
            n169 = stacked-sequence {
              tunnel: w248 -> [_ _ w302 _]
              tunnel: w250 -> [_ _ w301 _]
              tunnel: w251 -> [_ _ w300 _]
              frame #0 {
                # "Update Top Level (Cue)"
                n170 = local read "Cue Path"() -> (w253:path)
                n171 = Empty String/Path?(string/path=w253) -> (empty?=w257:bool)
                n172 = call <vilib>:"Check if File or Folder Exists.vi"("path"=w253) -> ("file or folder exists?"=w254:bool, "dup path"=w259:path)  [unwired: 8 in, 1 out]
                n173 = Not(x=w257) -> (.not. x?=w256:bool)
                n174 = And(x=w254, y=w256) -> (x .and. y?=w255:bool)
                n175 = case shown="False" w255 {
                  tunnel: w259 -> [_ w269]
                  frame False {
                    w260 = u32 0 ("List Cycles")
                    n176 = local read "Favorites"() -> (w266:T5)
                    n177 = Array Size(array=w266) -> (size(s)=w262:i32)
                    n178 = Random Number (0-1)() -> (number: 0 to 1=w265:dbl)
                    n179 = Decrement(x=w262) -> (x-1=w261:i32)
                    n180 = Multiply(x=w261, y=w265) -> (x*y=w268:dbl)
                    n181 = Index Array(array=w266, index=w268) -> (element=w267:T22)
                    n182 = Unbundle By Name(w267) -> ("Cue Path"=w264:path)
                    n183 = local write "List Cycles"(w260) -> ()
                    n184 = local write "Cycles"(w260) -> ()
                    n185 = One Button Dialog(message="Invalid path.\nLoading another path from the 'favorites' list") -> ()  [unwired: 1 in, 1 out]
                    n186 = local write "Cue Path"(w264) -> ()
                  }
                  frame True {
                    n187 = call "XMLtoQ.vi"("XML File Path"=w269) -> ("Cue out"=→"Actions":T8, "Description"=w274:T23)
                    n188 = File/Directory Info(path=w269) -> (last mod=→"Last Modified (when loaded)":timestamp, error out=→"error out":errorcluster)  [unwired: 1 in, 5 out]
                    n189 = Unbundle(w274) -> ("Cue Description"=→"Cue Description":string)  [unwired: 1 out]
                    n190 = local write "Stale"(FALSE ("Stale")) -> ()
                    "Active cue path" <- w269
                  }
                }
                n191 = local write "% completed"(0.0 ("% completed")) -> ()
              }
              frame #1 {
                # "Toggle = TRUE = Change Parameters\nToggle = FALSE = Run a Macro"
                # "Update Mid Level (Actions)"
                n192 = local read "Actions"() -> (w284:T8)
                n193 = local read "Cue Info"() -> (w283:T4)
                n194 = Index Array(array=w283) -> (element=w282:T24)  [unwired: 1 in]
                n195 = for {
                  tunnel: w284 -> [w298] mode=indexing
                  tunnel: [w297] -> w276 mode=indexing
                  tunnel: w282 -> [w296]
                  tunnel: "Macro deadtime (s)" -> [w294]
                  tunnel: "Params deadtime (s)" -> [w293]
                  tunnel: [w288] -> w281 mode=indexing
                  tunnel: [w285] -> w278 mode=concatenating
                  i -> [w287]
                  n196 = Unbundle By Name(w298) -> ("Comment"=w295:string, "Duration (s)"=w292:dbl, "Reps"=w286:i32, "Toggle"=w291:bool)
                  n197 = Bundle By Name(cluster=w296, "Action Description"=w295, "Duration (s)"=w292) -> (w297:T24)
                  n198 = Select(t=w293, s=w291, f=w294) -> (s? t:f=w290:dbl)
                  n199 = Add(x=w292, y=w290) -> (x+y=w289:dbl)
                  n200 = Initialize Array(w287, w286) -> (w285:i32[])
                  n201 = Multiply(x=w286, y=w289) -> (x*y=w288:dbl)
                }
                "RepAct#list" <- w278
                "Cue Info" <- w276
                n202 = Add Array Elements(numeric array=w281) -> (sum=→"Duration (s)":dbl)
              }
              frame #2 {
                # "Update Lower Level (Instructions)"
                n203 = local read "Actions"() -> (w304:T8)
                n204 = local read "Macro Info (display)"() -> (w306:T16)
                n205 = Index Array(array=w306) -> (element=w305:T25)  [unwired: 1 in]
                n206 = for {
                  tunnel: w305 -> [w315]
                  tunnel: [w314] -> w303 mode=indexing
                  tunnel: w304 -> [w313] mode=indexing
                  tunnel: [w312] -> w299 mode=indexing
                  shift-right: [w311] -> _
                  shift-left: w302 -> [w310]
                  tunnel: w301 -> [w309]
                  shift-right: [w308] -> _
                  shift-left: w300 -> [w307]
                  n207 = Unbundle By Name(w313) -> ("Toggle"=w316:bool)
                  n208 = case shown="False" w316 {
                    tunnel: w313 -> [w329 w364]
                    tunnel: [w319 w360] -> w314
                    tunnel: w315 -> [w325 w359]
                    tunnel: [w323 1] -> w312
                    tunnel: [w322 w357] -> w311
                    tunnel: w310 -> [w318 w357]
                    tunnel: w309 -> [w321 _]
                    tunnel: [w320 w356] -> w308
                    tunnel: w307 -> [_ w356]
                    frame False {
                      # "Macro"
                      n209 = Unbundle By Name(w329) -> ("Macro path"=w328:path)
                      n210 = call "XMLtoMacro.vi"("XML File Path"=w328) -> ("MacroSaveCluster"=w327:T26)
                      n211 = Unbundle By Name(w327) -> ("Changes"=w324:bool[][], "Instructions"=w326:T27)
                      n212 = for {
                        tunnel: w326 -> [w352] mode=indexing
                        tunnel: w325 -> [w351]
                        tunnel: [w350] -> w319 mode=indexing
                        tunnel: w324 -> [w334] mode=indexing
                        tunnel: [w346] -> w317
                        tunnel: w321 -> [w345]
                        tunnel: [w344] -> w320
                        shift-right: [w330] -> w322
                        shift-left: w318 -> [w331]
                        n213 = Unbundle By Name(w352) -> ("Duration"=w342:dbl, "Comment"=w343:string, "Output Bits"=w344:bool[], "Steps"=w349:i32, "Potentials"=w347:dbl[])
                        n214 = local read "Calibrations"() -> (w348:T6)
                        n215 = call "ApplyCalibration.vi"("Potentials"=w347, "# AO cards"=w345, "Calibrations"=w348) -> ("# always zero"=w346:i32, "Excitations"=w341:dbl[])  [unwired: 1 in]
                        n216 = call "SwapElectrodes.vi"("index 2"="iswap1_2", "index 1"="iswap1_1", "Excitations in"=w341) -> ("Excitations out"=w338:dbl[])
                        n217 = call "SwapElectrodes.vi"("index 2"="iswap2_2", "index 1"="iswap2_1", "Excitations in"=w338) -> ("Excitations out"=w335:dbl[])
                        n218 = Index Array(array=w334, index=1) -> (element=w332:bool)
                        n219 = Bundle By Name(cluster=w351, "Changes"=w334, "Duration (s)"=w342, "Instruction Description"=w343, "Output Bits"=w344, "Steps"=w349, "Excitations"=w335) -> (w350:T25)
                        n220 = Select(t=w335, s=w332, f=w331) -> (s? t:f=w330:dbl[])
                      }
                      "# always zero" <- w317
                      n221 = Array Size(array=w319) -> (size(s)=w323:i32)
                    }
                    frame True {
                      # "need to carry over excitations\neven for param changes\nbecause ToRAWcmds.vi\ndoesn't discriminate.\n\ndon't need to carry 'changes' or bits\nbecause execution loop does discriminate\n...carry outbits anyway, for display"
                      # "Parameters"
                      n222 = Unbundle By Name(w364) -> ("Duration (s)"=w363:dbl, "Comment"=w362:string)
                      n223 = Initialize Array(FALSE, 0 ("dimension size")) -> (w353:bool[])
                      n224 = Bundle By Name(cluster=w359, "Duration (s)"=w363, "Instruction Description"=w362, "Excitations"=w357, "Input Bits"=w353, "Output Bits"=w356) -> (w361:T25)
                      n225 = Build Array(w361) -> (w360:T29)
                    }
                  }
                }
                "Insts per Act" <- w299
                n226 = local write "Macro Info 2D"(w303) -> ()
              }
              frame #3 {
                # "Update display"
                n227 = local read "Actions"() -> (w369:T8)
                n228 = property on="Cue Info" class="Arr (strict)"() -> ("Index Values"=w368:u32[])  [unwired: 2 in, 2 out]
                n229 = Array Size(array=w369) -> (size(s)=w365:i32)
                n230 = Index Array(array=w368) -> (element=w366:u32)  [unwired: 1 in]
                n231 = Less?(x=w366, y=w365) -> (x < y?=w367:bool)
                n232 = case shown="True" w367 {
                  tunnel: w366 -> [_ w374]
                  frame False {
                  }
                  frame True {
                    n233 = Index Array(array="Macro Info 2D", index (row)=w374) -> (element=w375:T29)  [unwired: 1 in]
                    n234 = local read "# always zero"() -> (w373:i32)
                    n235 = local read "Calibrations"() -> (w372:T6)
                    n236 = for {
                      tunnel: w375 -> [w381] mode=indexing
                      tunnel: [w378] -> w370 mode=indexing
                      tunnel: w373 -> [w377]
                      tunnel: w372 -> [w376]
                      n237 = Unbundle By Name(w381) -> ("Excitations"=w379:dbl[])
                      n238 = call "RemoveCalibration.vi"("Excitations"=w379, "# always zero"=w377, "Calibrations"=w376) -> ("Potentials"=w380:dbl[])  [unwired: 2 in]
                      n239 = Bundle By Name(cluster=w381, "Excitations"=w380) -> (w378:T25)
                    }
                    "Macro Info (display)" <- w370
                  }
                }
              }
            }
          }
          frame "target stale" {
            n240 = local write "Target stale"(FALSE ("Value (Signaling)")) -> ()
            n241 = stacked-sequence {
              seq-local: [_ w404 _ _ _ _] -> [_ _ w415 _ _ _]
              seq-local: [_ w403 _ _ _ _] -> [_ _ w414 _ _ _]
              tunnel: [_ _ _ _ _ w495] -> w382
              frame #0 {
                # "double backslash because \\ is code"
                # "check that the cue matches the system selected on startup"
                n242 = local read "System"() -> (w390:u16)
                n243 = case shown="0, Default" w390 {
                  tunnel: ["CuspControl\\\\Positron" "CuspControl\\\\Musashi" "CuspControl\\\\Cusp"] -> w389
                  frame 1 {
                  }
                  frame 2 {
                  }
                  frame 0, Default {
                  }
                }
                n244 = local read "Cue Path"() -> (w391:path)
                n245 = Path To String(path=w391) -> (string=w388:string)
                n246 = Match Pattern(string=w388, regular expression=w389) -> (offset past match=w387:i32)  [unwired: 1 in, 3 out]
                n247 = Equal?(x=w387, y=-1) -> (x = y?=w385:bool)
                n248 = case shown="True" w385 {
                  tunnel: "Cue must match the system.\nSystem is set at startup, from the dropdown next to Stop VI.\nChange system (Cusp,Positron,Musashi) and start again." ("message") -> [_ w392]
                  frame False {
                  }
                  frame True {
                    n249 = One Button Dialog(message=w392, button name ("OK")="OK") -> (true=w394:bool)
                    n250 = Stop(stop? (T)=w394) -> ()
                  }
                }
              }
              frame #1 {
                # "If Variable Scan, update Actions or Macro Info 2D with new value"
                n251 = local read "Macro Info 2D"() -> (w401:T2)
                n252 = local read "Calibrations"() -> (w399:T6)
                n253 = local read "# always zero"() -> (w400:i32)
                n254 = local read "Actions"() -> (w402:T8)
                n255 = case shown="True" "Variable Scan" {
                  tunnel: [w405 w407] -> w404
                  tunnel: [w406 w408] -> w403
                  tunnel: w402 -> [w406 w411]
                  tunnel: w401 -> [w405 w412]
                  tunnel: w400 -> [_ w410]
                  tunnel: w399 -> [_ w409]
                  frame False {
                  }
                  frame True {
                    n256 = local read "Variable Cluster"() -> (w413:T17)
                    n257 = call "ParamScanSubVI.vi"("Variable Cluster"=w413, "Actions in"=w411, "Macro Info 2D in"=w412, "# always zero"=w410, "Calibrations"=w409) -> ("Actions out"=w408:T8, "Macro Info 2D out"=w407:T2)  [unwired: 5 in]
                    n258 = local write "Macro Info 2D"(w407) -> ()
                    n259 = local write "Actions"(w408) -> ()
                  }
                }
              }
              frame #2 {
                # "Convert all voltage ramps to RAW ramps (interleaved i16's)\nConvert Actions to RT format (Macros only, for now)"
                n260 = local write "Target stale"(TRUE ("Target stale")) -> ()
                n261 = local read "# AO cards"() -> (w420:u8)
                n262 = local read "Insts per Act"() -> (w418:i32[])
                n263 = call "ToRawCommands_RT.vi"("Macro Info 2D"=w415, "# AO cards"=w420) -> ("RAW cluster"=w419:cluster{i16[][]}[][])
                n264 = for {
                  tunnel: w415 -> [w427] mode=indexing
                  tunnel: w419 -> [w426] mode=indexing
                  tunnel: [w421] -> w417 mode=concatenating
                  tunnel: w418 -> [w425] mode=indexing
                  tunnel: w414 -> [w424] mode=indexing
                  n265 = Unbundle By Name(w424) -> ("Toggle"=w423:bool, "Reps"=w422:i32)
                  n266 = for {
                    N: w422 -> [_]
                    tunnel: w427 -> [w433]
                    tunnel: w426 -> [w432]
                    tunnel: w425 -> [w431]
                    tunnel: w423 -> [w429]
                    tunnel: [w428] -> w421 mode=indexing
                    n267 = call "ConvertAction.vi"("RAW cluster 2"=w432, "Macro Info 2D 2"=w433, "Instructions per Action"=w431) -> ("RT Action"=w430:T12)
                    n268 = Bundle(cluster=w430, "Toggle"=w429) -> (w428:T12)  [unwired: 3 in]
                  }
                }
                "RT Actions" <- w417
              }
              frame #3 {
                # "what actually happens in this cue"
                # "list of parameters and their attributes"
                # "start indices of parameter groups"
                # "Write slow AO (target) and txt (local) tables"
                n269 = local read "System"() -> (w450:u16)
                n270 = Index Array(array="Params paths", index=w450) -> (element=w455:path)
                n271 = Read from Text File(file (use dialog)=w455) -> (refnum out=w454:refnum<file>, text=w452:string, error out=w449:errorcluster)  [unwired: 3 in, 1 out]
                n272 = Initialize Array("") -> (w453:string[][])  [unwired: 2 in]
                n273 = Close File(refnum=w454, error in=w449) -> ()  [unwired: 2 out]
                n274 = Spreadsheet String To Array(format string="%s", spreadsheet string=w452, array type (2D Dbl)=w453) -> (array=w444:string[][])  [unwired: 1 in]
                n275 = Index Array(array=w444, index (col)=0 ("disabled index (col)")) -> (element=w448:string[])  [unwired: 1 in]
                n276 = for {
                  tunnel: w448 -> [w459] mode=indexing
                  shift-right: [w459] -> _
                  shift-left: "" -> [w458]
                  tunnel: [w456] -> w447 mode=indexing if=w457
                  tunnel: [w456] -> w439
                  i -> [w456]
                  n277 = Not Equal?(x=w458, y=w459) -> (x != y?=w457:bool)
                }
                n278 = Increment(x=w439) -> (x+1=w438:i32)
                n279 = local read "Actions"() -> (w446:T8)
                n280 = Build Array (concatenate)(w447, w438) -> (w445:i32[])
                n281 = local read "RT Actions"() -> (w441:T11)
                n282 = call "BuildParamSheet.vi"("StartParamIndices"=w445, "Params list"=w444, "Actions"=w446) -> ("DAC cmds"=w442:string[], "txt cmds"=→"Txt cmds":string[])
                n283 = call "AddSlowAO.vi"("RT Actions (without slowAO)"=w441, "DAC cmds"=w442) -> ("RT Actions"=w440:T12[])
                n284 = local write "RT Actions"(w440) -> ()
              }
              frame #4 {
                # "Send cue to RT target in bites that aren't too big for AMC"
                n285 = local read "RT Actions"() -> (w473:T11)
                n286 = Flatten To String(anything=w473) -> (data string=w472:string)  [unwired: 3 in, 2 out]
                n287 = local read "Target IP"() -> (w469:string)
                n288 = call "BreakupString.vi"("bite size"="bite size", "data string"=w472) -> ("Array"=w471:string[])
                n289 = local read "Target port"() -> (w465:u16)
                n290 = disable-structure shown="Enabled" {
                  disable-tunnel: [w475 w480] -> w463
                  disable-tunnel: [w474 errorcluster {"status"=FALSE, "code"=0, "source"=""} ("error out")] -> w461
                  frame Enabled {
                    n291 = local read "GUI_AMCname"() -> (w476:string)
                    n292 = call <vilib>:"Create Message Queue.vi"("message queue name"=w476) -> ("message queue out"=w475:T15, "error out"=w478:errorcluster)  [unwired: 13 in]
                    n293 = local read "Host port"() -> (w477:u16)
                    n294 = call <vilib>:"Start Dispatcher.vi"("UDP port (0)"=w477, "error in"=w478) -> ("error out"=w474:errorcluster)  [unwired: 11 in, 2 out]
                  }
                  frame Disabled {
                    n295 = local read "RT-to-GUI"() -> (w480:T15)
                  }
                }
                n296 = for {
                  tunnel: w465 -> [w494]
                  tunnel: w469 -> [w493]
                  tunnel: "RT Loop" ("receiver process") -> [w491]
                  tunnel: "New Cue" ("String") -> [w490]
                  shift-right: [w488] -> w460
                  shift-left: w461 -> [w492]
                  tunnel: w471 -> [w489] mode=indexing
                  n297 = call <vilib>:"Send Network Message.vi"("receiver process"=w491, "receiver host"=w493, "receiver port (0)"=w494, "message name"=w490, "message value"=w489, "error in"=w492) -> ("error out"=w488:errorcluster)  [unwired: 7 in, 2 out]
                  n298 = Wait (ms)(milliseconds to wait="milliseconds to wait") -> ()  [unwired: 1 out]
                }
                n299 = while {
                  tunnel: w463 -> [w486]
                  shift-right: [w484] -> w462
                  shift-left: w460 -> [w485]
                  stop <- w481 stop-if-true
                  n300 = call <vilib>:"Read Next Message.vi"("message queue in"=w486, "error in"=w485) -> ("message value"=w483:string, "error out"=w484:errorcluster)  [unwired: 6 in, 6 out]
                  n301 = Equal?(x="", y=w483) -> (x = y?=w481:bool)
                }
                n302 = local write "AMC error"(w462) -> ()
                n303 = Wait (ms)(milliseconds to wait=u32 500) -> ()  [unwired: 1 out]
                "Sending" <- TRUE ("Sending")
              }
              frame #5 {
                w497 = FALSE ("Target stale")
                # "autorun if var-scan"
                n304 = local read "Variable Scan"() -> (w496:bool)
                n305 = case shown="True" w496 {
                  tunnel: [State."idle" ("State") State."run" ("State")] -> w495
                  frame False {
                  }
                  frame True {
                  }
                }
                n306 = local write "Target stale"(w497) -> ()
                n307 = local write "Sending"(w497) -> ()
              }
            }
          }
          frame "run" {
            n308 = stacked-sequence {
              frame #0 {
                # "Write to log file; disable Run button until end of Cue"
                n309 = local read "Variable Cluster"() -> (w545:T17)
                n310 = local read "Cue Path"() -> (w541:path)
                n311 = Get Date/Time In Seconds() -> (seconds since 1Jan1904=w531:timestamp)
                n312 = Path To String(path=w541) -> (string=w538:string)
                n313 = Format Date/Time String(time format string (%c)="%H%M%S\\t", seconds (now)=w531) -> (date/time string=w527:string)  [unwired: 1 in]
                n314 = Unbundle By Name(w545) -> ("Variable Type"=w542:u16, "Values"=w544:dbl[], "Next Element"=w535:i32)  [unwired: 3 out]
                n315 = property on="Variable Type" class="Ring (strict)"() -> ("Strings []"=w543:string[])  [unwired: 2 in, 2 out]
                n316 = local read "Variable Scan"() -> (w537:bool)
                n317 = Concatenate Strings(w527, "Cue Path: %s" ("format string")) -> (w528:string)
                n318 = Index Array(array=w543, index=w542) -> (element=w540:string)
                n319 = Index Array(array=w544, index=w535) -> (element=w539:dbl)
                n320 = Concatenate Strings(w528, "\\tParameter: %s\\tValue: %e" ("format string")) -> (w536:string)
                n321 = Get Date/Time In Seconds() -> (seconds since 1Jan1904=w526:timestamp)
                n322 = case shown="True" w537 {
                  tunnel: w540 -> [_ w552]
                  tunnel: w539 -> [_ w551]
                  tunnel: w538 -> [w549 w555]
                  tunnel: [w550 w554] -> w533
                  tunnel: w536 -> [_ w553]
                  tunnel: w528 -> [w548 _]
                  frame False {
                    n323 = Format Into String(format string=w548, w549) -> (resulting string=w550:string)  [unwired: 2 in, 1 out]
                  }
                  frame True {
                    n324 = Format Into String(format string=w553, w555, w552, w551) -> (resulting string=w554:string)  [unwired: 2 in, 1 out]
                  }
                }
                n325 = Format Date/Time String(time format string (%c)="\\%Y-%m-%d.log", seconds (now)=w526) -> (date/time string=w524:string)  [unwired: 1 in]
                n326 = Path To String(path="Log Files path") -> (string=w525:string)
                n327 = Concatenate Strings(w525, w524) -> (w521:string)
                n328 = Concatenate Strings(w533, "\r\n") -> (w506:string)
                n329 = String To Path(string=w521) -> (path=w523:path)
                n330 = call <vilib>:"Check if File or Folder Exists.vi"("path"=w523) -> ("file or folder exists?"=w517:bool, "dup path"=w522:path)  [unwired: 8 in, 1 out]
                n331 = local read "Cycles"() -> (w503:u32)
                n332 = Select(t=T20."open" ("operation (0:open)"), s=w517, f=T20."create" ("operation (0:open)")) -> (s? t:f=w518:T20)
                n333 = property on="ABORT" class="Bool (strict)"("DisabledEnum"=T19."Enabled" ("Disabled")) -> ()  [unwired: 2 in, 2 out]
                n334 = Open/Create/Replace File(file path (use dialog)=w522, operation (0:open)=w518) -> (refnum out=w514:refnum<file>, error out=w513:errorcluster)  [unwired: 4 in, 1 out]
                n335 = Greater Than 0?(x=w503) -> (x > 0?=w504:bool)
                n336 = Read from Text File(file (use dialog)=w514, error in=w513) -> (refnum out=w516:refnum<file>, error out=w515:errorcluster)  [unwired: 2 in, 2 out]
                n337 = case shown="True" w504 {
                  tunnel: w503 -> [_ w546]
                  frame False {
                  }
                  frame True {
                    n338 = Decrement(x=w546) -> (x-1=w547:u32)
                    n339 = local write "Cycles"(w547) -> ()
                  }
                }
                n340 = Set File Position(refnum=w516, from (0:start)=enum16{"start", "end", "current"}."end", error in=w515) -> (refnum out=w512:refnum<file>, error out=w511:errorcluster)  [unwired: 1 in]
                n341 = Write to Text File(file (use dialog)=w512, text=w506, error in=w511) -> (refnum out=w519:refnum<file>, error out=w520:errorcluster)  [unwired: 1 in, 1 out]
                n342 = property on="Run" class="Bool (strict)"("DisabledEnum"=T19."Disabled" ("Disabled")) -> ()  [unwired: 2 in, 2 out]
                n343 = Close File(refnum=w519, error in=w520) -> ()  [unwired: 2 out]
              }
              frame #1 {
                # "Tell Target to run"
                n344 = disable-structure shown="Enabled" {
                  disable-tunnel: [w567 errorcluster {"status"=FALSE, "code"=0, "source"=""} ("error in")] -> w556
                  frame Enabled {
                    n345 = local read "GUI_AMCname"() -> (w566:string)
                    n346 = call <vilib>:"Create Message Queue.vi"("message queue name"=w566) -> ("error out"=w568:errorcluster)  [unwired: 13 in, 1 out]
                    n347 = local read "Host port"() -> (w565:u16)
                    n348 = call <vilib>:"Start Dispatcher.vi"("UDP port (0)"=w565, "error in"=w568) -> ("error out"=w567:errorcluster)  [unwired: 11 in, 2 out]
                  }
                  frame Disabled {
                  }
                }
                n349 = local read "Target port"() -> (w563:u16)
                n350 = local read "Target IP"() -> (w562:string)
                n351 = Flatten To String(anything=Request."Start" ("RT_State")) -> (data string=w558:string)  [unwired: 3 in, 2 out]
                n352 = call <vilib>:"Send Network Message.vi"("receiver process"="RT Loop", "receiver host"=w562, "receiver port (0)"=w563, "message name"="Run Control" ("String"), "message value"=w558, "error in"=w556) -> ("error out"=→"AMC error":errorcluster)  [unwired: 7 in, 2 out]
                n353 = Wait (ms)(milliseconds to wait=u32 100) -> ()  [unwired: 1 out]
              }
              frame #2 {
                w575 = 10000  # Max # of Actions
                # "Follow along with RT execution via AMC\nWrite text files when appropriate Action #'s are reached\nSend commands for interrupting or bypassing part of the Cue"
                n354 = local read "RepAct#list"() -> (w571:i32[])
                n355 = local read "Duration (s)"() -> (w579:dbl)
                n356 = local read "AMC error"() -> (w572:errorcluster)
                n357 = local read "Target port"() -> (w582:u16)
                n358 = local read "RT Actions"() -> (w583:T11)
                n359 = local read "RT-to-GUI"() -> (w570:T15)
                n360 = local read "Target IP"() -> (w581:string)
                n361 = local read "Txt cmds"() -> (w580:string[])
                n362 = Initialize Array(i64 0, w575) -> (w574:i64[])
                n363 = while {
                  tunnel: w583 -> [w603]
                  shift-right: [w600] -> w578
                  shift-left: w572 -> [w608]
                  tunnel: w570 -> [w611]
                  tunnel: w582 -> [w610]
                  tunnel: w581 -> [w609]
                  shift-right: [w605] -> w573
                  shift-left: -1 ("Action # out") -> [w607]
                  tunnel: w580 -> [w604]
                  tunnel: w579 -> [w599]
                  shift-right: [w596] -> _
                  shift-left: w574 -> [w597]
                  tunnel: w571 -> [w595]
                  stop <- w602 stop-if-true
                  n364 = Or(x="ABORT", y="Skip wait") -> (x .or. y?=w593:bool)
                  n365 = call "Comm.vi"("GUI Queue"=w611, "Target port"=w610, "Target IP"=w609, "Action # in"=w607, "Times in"=w597, "error in (no error)"=w608, "Skip wait"=w593) -> ("Next Action?"=w606:bool, "Action # out"=w605:i32, "Times out"=w596:i64[], "error out"=w601:errorcluster)  [unwired: 5 in]
                  n366 = Wait Until Next ms Multiple(millisecond multiple=u32 2) -> ()  [unwired: 1 out]
                  n367 = case shown="False" "Skip wait" {
                    frame False {
                    }
                    frame True {
                      n368 = local write "Skip wait"(FALSE ("Skip wait")) -> ()
                    }
                  }
                  n369 = case shown="False" w606 {
                    tunnel: w605 -> [w616 w625]
                    tunnel: w604 -> [_ w631]
                    tunnel: w603 -> [w618 w630]
                    tunnel: [w620 FALSE] -> w602
                    tunnel: w601 -> [w619 w633]
                    tunnel: [w619 w632] -> w600
                    tunnel: w599 -> [_ w629]
                    tunnel: w596 -> [_ w628]
                    tunnel: "ABORT" -> [w614 _]
                    tunnel: w595 -> [_ w624]
                    frame False {
                      # "continue until last action+1\nto get time of last action"
                      # "if no new action, check for end"
                      n370 = Array Size(array=w618) -> (size(s)=w617:i32)
                      n371 = Less Or Equal?(x=w617, y=w616) -> (x <= y?=w615:bool)
                      n372 = Or(x=w615, y=w614) -> (x .or. y?=w620:bool)
                    }
                    frame True {
                      w626 = i64 1000  # ms per s
                      n373 = call "WriteTextFiles.vi"("error in"=w633, "Action #"=w625, "RT Actions"=w630, "Txt cmds"=w631) -> ("error out"=w632:errorcluster)
                      n374 = Add Array Elements(numeric array=w628) -> (sum=w627:i64)
                      n375 = Index Array(array=w624, index=w625) -> (element=→"Current\nAction":i32)
                      n376 = Divide(x=w627, y=w626) -> (x/y=w623:dbl)
                      "Time (s)" <- w623
                      n377 = Divide(x=w623, y=w629) -> (x/y=→"% completed":dbl)
                      "Times (ms)" <- w628
                      "Timing" <- w628
                    }
                  }
                  n378 = case shown="False" "ABORT" {
                    selector: "ABORT" -> [_ w613]
                    frame False {
                    }
                    frame True {
                      n379 = local write "Zero All"(w613) -> ()
                    }
                  }
                }
                n380 = flat-sequence {
                  tunnel: w578 -> [w586]
                  tunnel: w573 -> [w590]
                  frame #0 {
                    n381 = local read "Timing"() -> (w591:i64[])
                    n382 = local write "AMC error"(w586) -> ()
                    n383 = local write "% completed"(1.0 ("% completed")) -> ()
                    n384 = Array Subset(array=w591, length=w590) -> (w589:i64[])  [unwired: 1 in]
                    n385 = local write "Run"(FALSE ("Execute")) -> ()
                    n386 = property on="Run" class="Bool (strict)"("DisabledEnum"=T19."Enabled" ("Disabled")) -> ()  [unwired: 2 in, 2 out]
                    n387 = property on="ABORT" class="Bool (strict)"("DisabledEnum"=T19."Disabled" ("Disabled")) -> ()  [unwired: 2 in, 2 out]
                    n388 = local write "Timing"(w589) -> ()
                  }
                }
              }
              frame #3 {
                # "This element of variable scan is done"
                n389 = local read "GUI-to-Scan"() -> (w636:T15)
                n390 = local write "Variable Scan"(FALSE ("Variable Scan")) -> ()
                n391 = call <vilib>:"Send Local Message.vi"("message queue in"=w636, "message name"="Done" ("Message Name")) -> ()  [unwired: 11 in, 3 out]
              }
            }
          }
          frame "zero all" {
            # "this command is sent directly to RT Loop\nwhen received, a 0 V cue replaces the cue previously in memory on target\ntarget proceeds to run that as soon as it finishes the last Action"
            n392 = flat-sequence {
              frame #0 {
                n393 = local read "error out"() -> (w640:errorcluster)
                n394 = local read "Target IP"() -> (w645:string)
                n395 = local read "Target port"() -> (w644:u16)
                n396 = call <vilib>:"Send Network Message.vi"("receiver process"="RT Loop", "receiver host"=w645, "receiver port (0)"=w644, "message name"="Zero All", "error in"=w640) -> ("error out"=w639:errorcluster)  [unwired: 8 in, 2 out]
                n397 = local write "error out"(w639) -> ()
                n398 = Wait (ms)(milliseconds to wait=u32 300) -> ()  [unwired: 1 out]
              }
              frame #1 {
                w647 = FALSE
                n399 = local write "Zero All"(w647) -> ()
                n400 = local write "Stale"(TRUE ("Target stale")) -> ()
                n401 = local write "ABORT"(w647) -> ()
                n402 = local write "Run"(w647) -> ()
              }
            }
          }
          frame "open cal" {
            n403 = flat-sequence {
              frame #0 {
                # "wait so that user\nsees that button was\npressed"
                n404 = Wait (ms)(milliseconds to wait=u32 100) -> ()  [unwired: 1 out]
              }
              frame #1 {
                n405 = local write "Open Calibration"(FALSE ("Save Calibration")) -> ()
                n406 = call "XMLtoCalibration.vi"("XML File Path"="Calibration path") -> ("Calibrations"=w653:T6)  [unwired: 1 in]
                n407 = local write "Stale"(TRUE ("Save Calibration")) -> ()
                n408 = local write "Calibrations"(w653) -> ()
              }
            }
          }
          frame "save cal" {
            n409 = local read "Calibration path"() -> (w657:path)
            n410 = local write "Save Calibration"(FALSE ("Save Calibration")) -> ()
            n411 = call "CalibrationtoXML.vi"("Calibrations"="Calibrations", "XML File Path"=w657) -> ()  [unwired: 1 out]
          }
        }
        "State" <- w101
        n412 = Wait (ms)(milliseconds to wait=u32 100) -> ()  [unwired: 1 out]
        n413 = Not(x="stop") -> (.not. x?=w104:bool)
      }
      n414 = local write "stop"(w99) -> ()
    }
    frame #2 {
      # "cleanup"
      n415 = local read "AMC error"() -> (w658:errorcluster)
      n416 = call <vilib>:"Stop Dispatcher.vi"("error in"=w658) -> ("error out"=w659:errorcluster)  [unwired: 14 in]
      n417 = property on="System" class="Ring (strict)"("DisabledEnum"=T19."Enabled" ("Disabled")) -> ()  [unwired: 2 in, 2 out]
      n418 = local write "AMC error"(w659) -> ()
    }
  }
